vi "CC Create Script.vi"(11 "script name in":string) -> (3 "script name out":string)   [LabVIEW 2024]
uses:
  typedefs/CC cluster Exposure.ctl
  Detector/Detector Class/Detector enum Detector Integration Mode.ctl
  typedefs/CC cluster sidereal rate.ctl
  typedefs/CC Dithering.ctl
  typedefs/CC cluster Offset Dithering.ctl
  typedefs/CC Dithering Offsets.ctl
  typedefs/cc cluster muRA muDEC.ctl
  typedefs/CC cluster Random Dithering.ctl
  Detector/FITS/FITS enum Data Type.ctl
  Telescope/CC cluster Telescope Offsets.ctl
  typedefs/CC cluster Object.ctl
  typedefs/CC cluster RA and DEC.ctl
  Telescope/Telescope cluster Equinox.ctl
  Telescope/Telescope cluster Parallax.ctl
  Telescope/Telescope cluster Rotator.ctl
  Telescope/Telesope ring Frame.ctl
  typedefs/CC Script Step.ctl
  typedefs/CC enum Script Action.ctl
  Scripts/CC Rd Wr Script Creator Defaults.ctl
  typedefs/CC Dithering Map.ctl
  typedefs/CC enum Dithering Types.ctl
  Detector/FITS/FITS cluster Header Row.ctl
  typedefs/CC cluster Script.ctl
  Subsystems/SS typedef cluster Instrument Command Queue Data.ctl
  Scripts/CC Rd Wr Script Action.ctl
  Focus/Focus cluster MoveFocus Command Parameters.ctl
  typedefs/CC cluster Outlet Control.ctl
  typedefs/CC cluster Filter Wheel Parameters.ctl
  typedefs/CC cluster Acquire Parameters.ctl
  typedefs/CC cluster Pause Parameters.ctl
  Filter Wheel/Filter Wheel Object/Filter Wheel.lvclass
  Telescope/Telescope.lvclass
panel:
  in  "Script Path":path
  in  "Delete":bool
  in  "New Button":bool
  in  "Save As Button":bool
  in  "Script Name":u16(ring) items=["FocusScan_20231229_125359", "FocusScan_20240105_105553", "FocusScan_20240105_111439", "FocusScan_20240105_113950", "FocusScan_20240105_114731", "FocusScan_20240105_114814", "FocusScan_20240105_114924", "FocusScan_20240105_120012", "FocusScan_20240503_180609", "FocusScan_20240508_153210", "FocusScan_20240508_155921", "FocusScan_20240508_162716", "FocusScan_20240508_163450", "FocusScan_20240523_232945", "FocusScan_20240524_142601", "FocusScan_20240524_144640", "FocusScan_20240528_161613", "FocusScan_20240528_162302", "FocusScan_20240528_171448", "FocusScan_20240805_154542", "FocusScan_20240805_160317", "joe_test", "Obs_", "Obs_A00098", "Obs_A00099", "Obs_A00100", "Obs_A00101", "Obs_A00102", "Obs_A00103", "Obs_A00104", "Obs_A00105", "Obs_A00106", "Obs_A00107", "Obs_A00108", "Obs_A00109", "Obs_A00110", "Obs_A00111", "Obs_A00112", "Obs_A00113", "Obs_A00114", "Obs_A00115", "Obs_P00006", "Obs_P00008", "Obs_P00013", "Obs_P00014", "Obs_P00017", "Obs_P00018", "Obs_P00020", "Obs_P00022", "Obs_P00024", "Obs_P00025", "Obs_P00028", "Obs_P00033", "Obs_P00036", "Obs_P00037", "Obs_P00039", "Obs_P00040", "Obs_P00041", "Obs_P00042", "Obs_P00043", "Obs_P00044", "Obs_P00045", "Obs_P00046", "Obs_P00047", "Obs_P00049", "Obs_P00050", "Obs_P00051", "Obs_P00052", "Obs_P00053", "Obs_P00054", "Obs_P00055", "Obs_P00058", "Obs_P00059", "Obs_P00061", "Obs_P00064", "Obs_P00066", "Obs_P00067", "Obs_P00068", "Obs_P00069", "Obs_P00070", "Obs_P00071", "Obs_P00072", "Obs_P00073", "Obs_P00074", "Obs_P00075", "Obs_P00077", "Obs_P00078", "Obs_P00079", "Obs_P00080", "Obs_P00082", "Obs_P00083", "Obs_P00084", "Obs_P00085", "Obs_P00089", "Obs_P00090", "Obs_P00091", "Obs_P00092", "Obs_P00093", "Obs_P00094", "Obs_P00098", "Obs_P00099", "Obs_P00100", "Obs_P00101", "Obs_P00102", "Obs_P00103", "Obs_P00104", "Obs_P00105", "Obs_P00106", "Obs_P00107", "Obs_P00108", "Obs_P00109", "Obs_P00110", "Obs_P00111", "Obs_P00112", "Obs_P00113", "Obs_P00114", "Obs_P00115", "Obs_P00116", "Obs_P00117", "Obs_P00118", "Obs_P00119", "Obs_P00120", "Obs_P00121", "Obs_P00122", "Obs_P00123", "Obs_P00128", "Obs_P00129", "Obs_P00132", "Obs_P00133", "Obs_P00134", "Obs_P00135", "Obs_P00136", "Obs_P00137", "Obs_P00138", "Obs_P00139", "Obs_P00141", "Obs_P00142", "Obs_P00143", "Obs_P00144", "Obs_P00145", "Obs_P00146", "Obs_P00147", "Obs_P00148", "Obs_P00149", "Obs_P00150", "Obs_P00151", "Obs_P00152", "Obs_P00153", "Obs_P00162", "Obs_P00163", "Obs_P00164", "Obs_P00165", "Obs_P00166", "Obs_P00167", "Obs_P00168", "Obs_P00169", "Obs_P00170", "Obs_P00171", "Obs_P00172", "Obs_P00173", "Obs_P00174", "Obs_P00175", "Obs_P00176", "Obs_P00177", "Obs_P00178", "Obs_P00179", "Obs_P00180", "Obs_P00181", "Obs_P00182", "Obs_P00183", "Obs_P00184", "Obs_P00185", "Obs_P00186", "Obs_P00187", "Obs_P00188", "Obs_P00189", "Obs_P00190", "Obs_P00191", "Obs_P00192", "Obs_P00193", "Obs_P00194", "Obs_P00195", "Obs_P00196", "Obs_P00197", "Obs_P00198", "Obs_P00286", "Obs_P00287", "Obs_P00386", "Obs_P00387", "Obs_P00466", "Obs_P00467", "Obs_P00566", "Obs_P00567", "Obs_P00666", "Obs_P00667", "Obs_P00746", "Obs_P00747", "Obs_P00846", "Obs_P00847", "Obs_P00946", "Obs_P00947", "Obs_P01069", "Obs_P01070", "Obs_P01071", "Obs_P01666", "Obs_P01667", "power_test", "QuickObs_20231204_145334", "QuickObs_20231204_153100", "QuickObs_20231204_154938", "QuickObs_20231204_155404", "QuickObs_20231205_121758", "QuickObs_20240223_111256", "QuickObs_20240223_111314", "QuickObs_20240223_111324", "QuickObs_20240223_133303", "QuickObs_20240223_134117", "QuickObs_20240223_134543", "QuickObs_20240223_140340", "QuickObs_20240229_123536", "QuickObs_20240301_132858", "QuickObs_20240508_165728", "QuickObs_20240509_165826", "QuickObs_20240513_000104", "QuickObs_20240521_153751", "QuickObs_20240523_163529", "QuickObs_20240523_164254", "QuickObs_20240523_164316", "QuickObs_20240523_164354", "QuickObs_20240523_164558", "QuickObs_20240523_164836", "QuickObs_20240523_164937", "QuickObs_20240523_230241", "QuickObs_20240528_161057", "QuickObs_20240528_161742", "QuickObs_20240528_174732", "QuickObs_20240531_164244", "QuickObs_20240531_170220", "QuickObs_20240531_171735", "QuickObs_20240531_172457", "QuickObs_20240531_172609", "QuickObs_20240531_173041", "QuickObs_20240603_173837", "QuickObs_20240603_180156", "QuickObs_20240603_181309", "QuickObs_20240603_181617", "QuickObs_20240603_181820", "QuickObs_20240603_182118", "QuickObs_20240603_182553", "QuickObs_20240603_222300", "QuickObs_20240603_222614", "QuickObs_20240603_223000", "QuickObs_20240603_223344", "QuickObs_20240603_223915", "QuickObs_20240627_110641", "QuickObs_20240814_205941", "QuickObs_20240821_123647", "QuickObs_20240821_124152", "QuickObs_20240821_124547", "QuickObs_20240822_145236", "QuickObs_20240822_150150", "QuickObs_20240822_150414", "QuickObs_20240822_150607", "QuickObs_20240822_151545", "QuickObs_20240822_151844", "QuickObs_20240822_152439", "QuickObs_20240822_153207", "QuickObs_20240822_160035", "QuickObs_20240822_160608", "QuickObs_20240822_161129", "QuickObs_20240822_162300", "QuickObs_20240823_115930", "QuickObs_20240823_164127", "QuickObs_20240903_141058", "QuickObs_20240903_144343", "QuickObs_20240903_144643", "QuickObs_20240903_144654", "QuickObs_20240903_152244", "QuickObs_20240903_152705", "QuickObs_20240903_152922", "QuickObs_20240905_141101", "QuickObs_20240905_141629", "QuickObs_20240906_143746", "QuickObs_20240906_144857", "QuickObs_20240906_150256", "QuickObs_20240906_151102", "QuickObs_20240906_153044", "QuickObs_20240906_153745", "QuickObs_20240906_155352", "QuickObs_20240906_160445", "QuickObs_20240906_160908", "QuickObs_20240906_162122", "QuickObs_20240906_163123", "QuickObs_20240909_133034", "QuickObs_20240909_133716", "QuickObs_20240909_134628", "QuickObs_20240909_154242", "QuickObs_20240909_154542", "QuickObs_20240909_154633", "QuickObs_20240909_154947", "QuickObs_20240909_155344", "QuickObs_20240909_155456", "QuickObs_20240909_161838", "QuickObs_20240909_162303", "QuickObs_20240909_162501", "QuickObs_20240909_162628", "QuickObs_20240909_163134", "QuickObs_20240909_163322", "QuickObs_20240909_163424", "QuickObs_20240909_163636", "QuickObs_20240909_163836", "QuickObs_20240909_164419", "QuickObs_20240909_170410", "QuickObs_20240909_170734", "QuickObs_20240909_171023", "QuickObs_20240909_171530", "QuickObs_20240909_172951", "QuickObs_20240909_173144", "QuickObs_20240909_173940", "QuickObs_20240909_174042", "QuickObs_20240909_174245", "QuickObs_20240909_174431", "QuickObs_20240909_175227", "QuickObs_20240909_175352", "QuickObs_20240909_175611", "QuickObs_20240909_181046", "QuickObs_20240909_181216", "QuickObs_20240909_181334", "QuickObs_20240909_181505", "QuickObs_20240909_181623", "QuickObs_20240909_181711", "QuickObs_20240910_131018", "QuickObs_20240910_131144", "QuickObs_20240910_131417", "QuickObs_20240910_131600", "QuickObs_20240910_132017", "QuickObs_20240910_132419", "QuickObs_20240910_160952", "QuickObs_20240910_161811", "QuickObs_20240910_162606", "QuickObs_20240910_162747", "QuickObs_20240910_163442", "QuickObs_20240910_163715", "QuickObs_20240910_164302", "QuickObs_20240910_164445", "QuickObs_20240910_164629", "QuickObs_20240910_165143", "QuickObs_20240910_165430", "QuickObs_20240910_165827", "QuickObs_20240910_170042", "QuickObs_20240910_171946", "QuickObs_20240910_172143", "QuickObs_20240910_172830", "QuickObs_20240910_173047", "QuickObs_20240910_173807", "QuickObs_20240910_173956", "QuickObs_20240912_161641", "QuickObs_20240912_161849", "QuickObs_20240912_162058", "QuickObs_20240912_163325", "QuickObs_20240913_112043", "QuickObs_20240913_112810", "QuickObs_20240913_113523", "QuickObs_20240913_113948", "QuickObs_20240913_115247", "QuickObs_20240913_115435", "QuickObs_20240913_120048", "QuickObs_20240913_120152", "random", "Test Focus", "TestCommandLine"]
  in  "Save Script":bool
  in  "Close":bool
  in  "Script":i32(listbox)
  in  "Tab Control":T1(tab)
  in  "Units":string
  in  "Open Button":bool
  out "FITS Header Template":path
  in  "Save Header":bool
  in  "Add/Replace":bool
  in  "Comment":string
  in  "Value":string
  in  "Header Field":string(combo)
  in  "FITS Header":i32(listbox)
  in  "Type":T2
  in  "RA and DEC String":cluster{"RA":string, "DEC":string}={"RA"="HH:MM:SS.nnn", "DEC"="DEG:arcmin:arcsec.nn"} caption="RA and DEC"
  in  "Obj Add to Script":bool
  in  "Obj Remove":bool
  in  "Object Name":cluster{"Name":string}
  in  "Sidereal Rate":T3
  in  "Obj Add/Replace":bool
  in  "Objects":i32(listbox)
  in  "Proper Motion":T4
  in  "Offsets":T5
  in  "Exp Add to Script":bool
  in  "Exp Remove":bool
  in  "Exp Add/Replace":bool
  in  "Exposure":T6={"Mode"=enum."CDS", "Integration Time"=1.0, "Name"="", "Images"=1}
  in  "Exposures":i32(listbox)
  in  "Add FW 4":bool
  in  "Add FW 3":bool
  in  "Add FW 2":bool
  in  "Add FW 1":bool
  in  "Filter Wheel 4":i32(listbox)
  in  "Filter Wheel 3":i32(listbox)
  in  "Filter Wheel 2":i32(listbox) caption="FW HK"
  in  "Filter Wheel 1":i32(listbox) caption="FW YJ"
  in  "Name":string
  in  "Dither Add to Script":bool
  in  "Dithering Add/Replace":bool
  in  "Dithering":i32(listbox)
  in  "Dithering Remove":bool
  in  "Dither Select":enum32{"Random", "Offset"}(tab)
  in  "Random Dither":T8={"Count"=1, "Radius"=1.0, "Name"=""}
  in  "Dithering Offset":T9
  in  "Add Image Acq":bool
  in  "Acquire Parameters":T12
  in  "Add Macro":bool
  in  "Script to Call":u16(ring) items=["FocusScan_20231229_125359", "FocusScan_20240105_105553", "FocusScan_20240105_111439", "FocusScan_20240105_113950", "FocusScan_20240105_114731", "FocusScan_20240105_114814", "FocusScan_20240105_114924", "FocusScan_20240105_120012", "FocusScan_20240503_180609", "FocusScan_20240508_153210", "FocusScan_20240508_155921", "FocusScan_20240508_162716", "FocusScan_20240508_163450", "FocusScan_20240523_232945", "FocusScan_20240524_142601", "FocusScan_20240524_144640", "FocusScan_20240528_161613", "FocusScan_20240528_162302", "FocusScan_20240528_171448", "FocusScan_20240805_154542", "FocusScan_20240805_160317", "joe_test", "Obs_", "Obs_A00098", "Obs_A00099", "Obs_A00100", "Obs_A00101", "Obs_A00102", "Obs_A00103", "Obs_A00104", "Obs_A00105", "Obs_A00106", "Obs_A00107", "Obs_A00108", "Obs_A00109", "Obs_A00110", "Obs_A00111", "Obs_A00112", "Obs_A00113", "Obs_A00114", "Obs_A00115", "Obs_P00006", "Obs_P00008", "Obs_P00013", "Obs_P00014", "Obs_P00017", "Obs_P00018", "Obs_P00020", "Obs_P00022", "Obs_P00024", "Obs_P00025", "Obs_P00028", "Obs_P00033", "Obs_P00036", "Obs_P00037", "Obs_P00039", "Obs_P00040", "Obs_P00041", "Obs_P00042", "Obs_P00043", "Obs_P00044", "Obs_P00045", "Obs_P00046", "Obs_P00047", "Obs_P00049", "Obs_P00050", "Obs_P00051", "Obs_P00052", "Obs_P00053", "Obs_P00054", "Obs_P00055", "Obs_P00058", "Obs_P00059", "Obs_P00061", "Obs_P00064", "Obs_P00066", "Obs_P00067", "Obs_P00068", "Obs_P00069", "Obs_P00070", "Obs_P00071", "Obs_P00072", "Obs_P00073", "Obs_P00074", "Obs_P00075", "Obs_P00077", "Obs_P00078", "Obs_P00079", "Obs_P00080", "Obs_P00082", "Obs_P00083", "Obs_P00084", "Obs_P00085", "Obs_P00089", "Obs_P00090", "Obs_P00091", "Obs_P00092", "Obs_P00093", "Obs_P00094", "Obs_P00098", "Obs_P00099", "Obs_P00100", "Obs_P00101", "Obs_P00102", "Obs_P00103", "Obs_P00104", "Obs_P00105", "Obs_P00106", "Obs_P00107", "Obs_P00108", "Obs_P00109", "Obs_P00110", "Obs_P00111", "Obs_P00112", "Obs_P00113", "Obs_P00114", "Obs_P00115", "Obs_P00116", "Obs_P00117", "Obs_P00118", "Obs_P00119", "Obs_P00120", "Obs_P00121", "Obs_P00122", "Obs_P00123", "Obs_P00128", "Obs_P00129", "Obs_P00132", "Obs_P00133", "Obs_P00134", "Obs_P00135", "Obs_P00136", "Obs_P00137", "Obs_P00138", "Obs_P00139", "Obs_P00141", "Obs_P00142", "Obs_P00143", "Obs_P00144", "Obs_P00145", "Obs_P00146", "Obs_P00147", "Obs_P00148", "Obs_P00149", "Obs_P00150", "Obs_P00151", "Obs_P00152", "Obs_P00153", "Obs_P00162", "Obs_P00163", "Obs_P00164", "Obs_P00165", "Obs_P00166", "Obs_P00167", "Obs_P00168", "Obs_P00169", "Obs_P00170", "Obs_P00171", "Obs_P00172", "Obs_P00173", "Obs_P00174", "Obs_P00175", "Obs_P00176", "Obs_P00177", "Obs_P00178", "Obs_P00179", "Obs_P00180", "Obs_P00181", "Obs_P00182", "Obs_P00183", "Obs_P00184", "Obs_P00185", "Obs_P00186", "Obs_P00187", "Obs_P00188", "Obs_P00189", "Obs_P00190", "Obs_P00191", "Obs_P00192", "Obs_P00193", "Obs_P00194", "Obs_P00195", "Obs_P00196", "Obs_P00197", "Obs_P00198", "Obs_P00286", "Obs_P00287", "Obs_P00386", "Obs_P00387", "Obs_P00466", "Obs_P00467", "Obs_P00566", "Obs_P00567", "Obs_P00666", "Obs_P00667", "Obs_P00746", "Obs_P00747", "Obs_P00846", "Obs_P00847", "Obs_P00946", "Obs_P00947", "Obs_P01069", "Obs_P01070", "Obs_P01071", "Obs_P01666", "Obs_P01667", "power_test", "QuickObs_20231204_145334", "QuickObs_20231204_153100", "QuickObs_20231204_154938", "QuickObs_20231204_155404", "QuickObs_20231205_121758", "QuickObs_20240223_111256", "QuickObs_20240223_111314", "QuickObs_20240223_111324", "QuickObs_20240223_133303", "QuickObs_20240223_134117", "QuickObs_20240223_134543", "QuickObs_20240223_140340", "QuickObs_20240229_123536", "QuickObs_20240301_132858", "QuickObs_20240508_165728", "QuickObs_20240509_165826", "QuickObs_20240513_000104", "QuickObs_20240521_153751", "QuickObs_20240523_163529", "QuickObs_20240523_164254", "QuickObs_20240523_164316", "QuickObs_20240523_164354", "QuickObs_20240523_164558", "QuickObs_20240523_164836", "QuickObs_20240523_164937", "QuickObs_20240523_230241", "QuickObs_20240528_161057", "QuickObs_20240528_161742", "QuickObs_20240528_174732", "QuickObs_20240531_164244", "QuickObs_20240531_170220", "QuickObs_20240531_171735", "QuickObs_20240531_172457", "QuickObs_20240531_172609", "QuickObs_20240531_173041", "QuickObs_20240603_173837", "QuickObs_20240603_180156", "QuickObs_20240603_181309", "QuickObs_20240603_181617", "QuickObs_20240603_181820", "QuickObs_20240603_182118", "QuickObs_20240603_182553", "QuickObs_20240603_222300", "QuickObs_20240603_222614", "QuickObs_20240603_223000", "QuickObs_20240603_223344", "QuickObs_20240603_223915", "QuickObs_20240627_110641", "QuickObs_20240814_205941", "QuickObs_20240821_123647", "QuickObs_20240821_124152", "QuickObs_20240821_124547", "QuickObs_20240822_145236", "QuickObs_20240822_150150", "QuickObs_20240822_150414", "QuickObs_20240822_150607", "QuickObs_20240822_151545", "QuickObs_20240822_151844", "QuickObs_20240822_152439", "QuickObs_20240822_153207", "QuickObs_20240822_160035", "QuickObs_20240822_160608", "QuickObs_20240822_161129", "QuickObs_20240822_162300", "QuickObs_20240823_115930", "QuickObs_20240823_164127", "QuickObs_20240903_141058", "QuickObs_20240903_144343", "QuickObs_20240903_144643", "QuickObs_20240903_144654", "QuickObs_20240903_152244", "QuickObs_20240903_152705", "QuickObs_20240905_141101", "QuickObs_20240905_141629", "QuickObs_20240906_143746", "QuickObs_20240906_144857", "QuickObs_20240906_150256", "QuickObs_20240906_151102", "QuickObs_20240906_153044", "QuickObs_20240906_153745", "QuickObs_20240906_155352", "QuickObs_20240906_160445", "QuickObs_20240906_160908", "QuickObs_20240906_162122", "QuickObs_20240906_163123", "QuickObs_20240909_133034", "QuickObs_20240909_133716", "QuickObs_20240909_134628", "QuickObs_20240909_154242", "QuickObs_20240909_154542", "QuickObs_20240909_154633", "QuickObs_20240909_154947", "QuickObs_20240909_155344", "QuickObs_20240909_155456", "QuickObs_20240909_161838", "QuickObs_20240909_162303", "QuickObs_20240909_162501", "QuickObs_20240909_162628", "QuickObs_20240909_163134", "QuickObs_20240909_163322", "QuickObs_20240909_163424", "QuickObs_20240909_163636", "QuickObs_20240909_163836", "QuickObs_20240909_164419", "QuickObs_20240909_170410", "QuickObs_20240909_170734", "QuickObs_20240909_171023", "QuickObs_20240909_171530", "QuickObs_20240909_172951", "QuickObs_20240909_173144", "QuickObs_20240909_173940", "QuickObs_20240909_174042", "QuickObs_20240909_174245", "QuickObs_20240909_174431", "QuickObs_20240909_175227", "QuickObs_20240909_175352", "QuickObs_20240909_175611", "QuickObs_20240909_181046", "QuickObs_20240909_181216", "QuickObs_20240909_181334", "QuickObs_20240909_181505", "QuickObs_20240909_181623", "QuickObs_20240909_181711", "QuickObs_20240910_131018", "QuickObs_20240910_131144", "QuickObs_20240910_131417", "QuickObs_20240910_131600", "QuickObs_20240910_132017", "QuickObs_20240910_132419", "QuickObs_20240910_160952", "QuickObs_20240910_161811", "QuickObs_20240910_162606", "QuickObs_20240910_162747", "QuickObs_20240910_163442", "QuickObs_20240910_163715", "QuickObs_20240910_164302", "QuickObs_20240910_164445", "QuickObs_20240910_164629", "QuickObs_20240910_165143", "QuickObs_20240910_165430", "QuickObs_20240910_165827", "QuickObs_20240910_170042", "QuickObs_20240910_171946", "QuickObs_20240910_172143", "QuickObs_20240910_172830", "QuickObs_20240910_173047", "QuickObs_20240910_173807", "QuickObs_20240910_173956", "QuickObs_20240912_161641", "QuickObs_20240912_161849", "QuickObs_20240912_162058", "QuickObs_20240912_163325", "QuickObs_20240913_112043", "QuickObs_20240913_112810", "QuickObs_20240913_113523", "QuickObs_20240913_113948", "QuickObs_20240913_115247", "QuickObs_20240913_115435", "QuickObs_20240913_120048", "QuickObs_20240913_120152", "random", "Test Focus", "TestCommandLine"]
  in  "Move Telescope":bool
  in  "RA and DEC String 2":cluster{"RA":string, "DEC":string}={"RA"="HH:MM:SS.nnn", "DEC"="DEG:arcmin:arcsec.nn"} caption="RA and DEC"
  in  "Telescope Focus":T13
  in  "Message for User":string
  in  "Add Ask":bool caption="Add Ask to Script"
  in  "Seconds to Pause":dbl=10.0
  in  "Add Pause":bool caption="Add Pause to Script"
  in  "Home Focus":bool
  in  "Absolute":bool
  in  "Relative":bool
  in  "Steps":i32
  in  "Select Motor (0:n-1)":i32 min=0 max=3 step=1
  in  "Add Outlet Cmd":bool caption="Add Outlet Command Step"
  in  "Outlet State":bool
  in  "Outlet Index (0 based)":i32
  in  "Add CmdLine":bool caption="Add CmdLine to Script"
  in  "Command Line":string
  in  "Add No-op":bool caption="Add Noop to Script"
  out "Script As Text":string="DefineObject Alpha1234 Standard RA=123.456 DEC=456.789\nDefineExposure Number=1,Groups=1,ReadoutsPerGroup=1,TimeBetweenGroups=10,TimeBetweenReadouts=10\nDefineDithering DEC=0,-10,+10 RA=0,-10,+10\nMoveFilter A,B\nAcquireImages [This command acquires image at every dithering position]\n\n"
  in  "Send":bool
  in  "Script Line":string
  # "Select a Configuration (PRIME or RIMAS, FilterWheel, etc.)"
  # "\"\t   Y, J, or H can go with Open or Narrow only\n\"\t  Z must go with Open\n\"\t Dark can go with anything\n\"\t Open can go with anything\n\"\t Narrow can only go with T, J, H"
  # "arcseconds"
  # "arcseconds"
  # "Telescope Pointing"
  # "Focus"
  # "The noop command is used for testing purposes. There are no parameters."
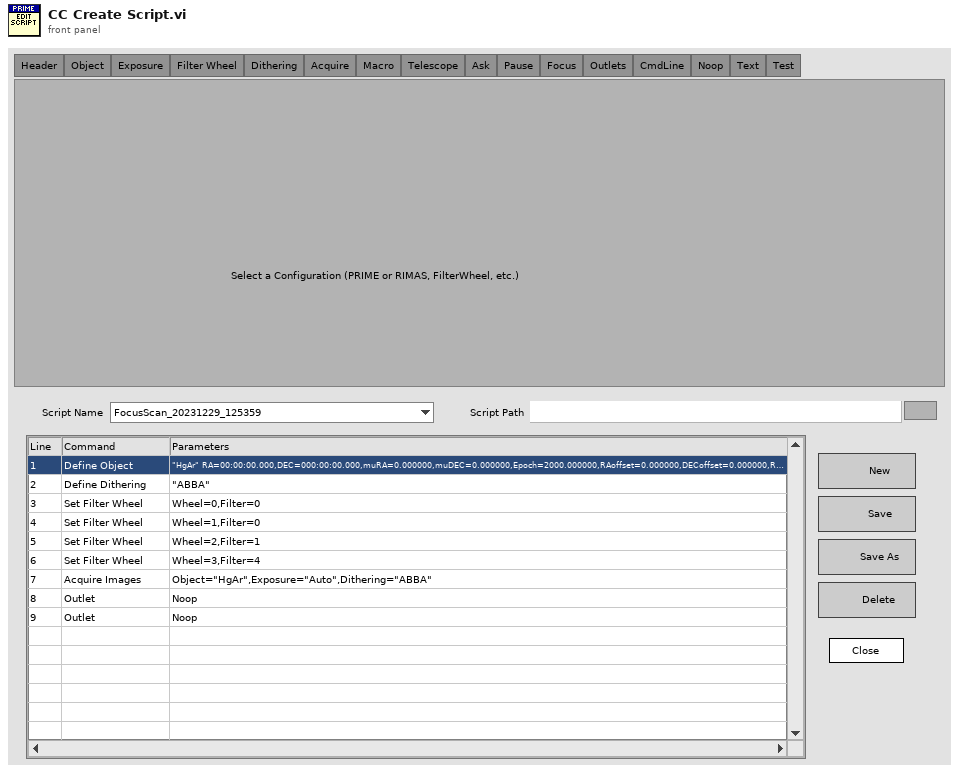
[diagram p1: front panel]
types:
  T1 = enum32{"Setup", "Header", "Object", "Exposure", "Filter Wheel", "Dithering", "Acquire", "Macro", "Telescope", "Ask", "Pause", "Focus", "Outlets", "CmdLine", "Noop", "Text", "Test"}
  T2 = typedef "FITS enum Data Type.ctl" = enum16{"String", "Integer", "Float"}
  T3 = typedef "CC cluster sidereal rate.ctl" = cluster{"dRA":dbl, "dDEC":dbl}
  T4 = typedef "cc cluster muRA muDEC.ctl" = cluster{"muRA":dbl, "muDEC":dbl, "Epoch":dbl}
  T5 = typedef "CC cluster Telescope Offsets.ctl" = cluster{"RA":dbl, "DEC":dbl, "ROT":dbl}
  T6 = typedef "CC cluster Exposure.ctl" = cluster{"Mode":T7, "Integration Time":dbl, "Name":string, "Images":i32}
  T7 = typedef "Detector enum Detector Integration Mode.ctl" = enum16{"Ramp", "CDS", "FOWLER2", "FOWLER4", "FOWLER8", "FOWLER16", "Raw"}
  T8 = typedef "CC cluster Random Dithering.ctl" = cluster{"Count":i32, "Radius":dbl, "Name":string}
  T9 = typedef "CC Dithering.ctl" = cluster{"Name":string, "Dithering Offsets":T10}
  T10 = typedef "CC cluster Offset Dithering.ctl" = cluster{"Offsets":T11[]}
  T11 = typedef "CC Dithering Offsets.ctl" = cluster{"DEC":dbl, "RA":dbl}
  T12 = cluster{"Object":string, "Exposure":string, "Dithering":string}
  T13 = cluster{"Focus Home":bool, "Move Focus":bool, "Position":dbl}
  T14 = typedef "CC cluster Object.ctl" = cluster{"Object":cluster{"Name":string}, "Sidereal Rate":T3, "RA and DEC":T15, "Proper Motion":T4, "Offsets":T5, "Equinox":T16, "Parallax":T17, "Rotator":T18, "Frame":T19, "Frac Rate":dbl, "Wavelength":dbl}
  T15 = typedef "CC cluster RA and DEC.ctl" = cluster{"RA":dbl, "DEC":dbl}
  T16 = typedef "Telescope cluster Equinox.ctl" = cluster{"Equinox Year":i32, "Equinox Prefix":string}
  T17 = typedef "Telescope cluster Parallax.ctl" = cluster{"Parallax":dbl, "rv kps":dbl}
  T18 = typedef "Telescope cluster Rotator.ctl" = cluster{"Frame":string, "PA":dbl}
  T19 = typedef "Telesope ring Frame.ctl" = enum16{"FK4", "FK5", "APPT", "GAPPT", "AZEL"}
  T20 = typedef "CC Script Step.ctl" = cluster{"Action":T21, "Data":variant}
  T21 = typedef "CC enum Script Action.ctl" = enum16{"Noop", "Define Object", "Define Exposure", "Define Dithering", "Acquire Images", "Set Filter Wheel", "Telescope Home", "Telescope Move", "Telescope RA DEC", "Focus Move Relative", "Focus Move Absolute", "Focus Set Home", "Macro", "Pause", "Ask User", "Define Random Dither", "CmdLine", "Outlet"}
  T22 = typedef "CC Rd Wr Script Creator Defaults.ctl" = cluster{"Script":string, "Script Path":path}
  T23 = typedef "CC Dithering Map.ctl" = cluster{"Name":string, "Dithering Offsets":T9, "Dithering Type":T24, "Random Dither":T8}
  T24 = typedef "CC enum Dithering Types.ctl" = enum16{"Random", "Offsets", "None"}
  T25 = typedef "FITS cluster Header Row.ctl" = cluster{"Field Name":string, "Type":T2, "Value":string, "Comment":string, "Units":string}
  T26 = cluster{"state":refnum<user-event>, "Object Map":map{string, T14}, "curr object":string, "Exp Map":map{string, T6}, "Script":T20[], "Settings":T22, "test":T20[], "Dither Map":map{string, T23}, "Hdr Map":map{string, T25}}
  T27 = typedef "CC cluster Script.ctl" = cluster{"Name":string, "Script":T20[]}
  T28 = typedef "CC Rd Wr Script Action.ctl" = enum16{"Read", "Write", "List", "Delete"}
  T29 = typedef "SS typedef cluster Instrument Command Queue Data.ctl" = cluster{"Cmd":string, "Parameters":variant}
  T30 = typedef "Focus cluster MoveFocus Command Parameters.ctl" = cluster{"Motor":i32, "Position":i32}
  T31 = typedef "CC cluster Outlet Control.ctl" = cluster{"Outlet Idx":i32, "State":bool}
  T32 = typedef "CC cluster Filter Wheel Parameters.ctl" = cluster{"Wheel":i32, "Filter":i32}
  T33 = enum32{"Setup", "Object", "Exposure", "Dithering", "Acquire", "Filter Wheel", "Focus", "Macro", "Ask", "Pause", "Noop", "Text", "Test"}
  T34 = enum32{"Setup", "Object", "Exposure", "Dithering", "Acquire", "Filter Wheel", "Focus", "Ask", "Pause", "Noop", "Text", "Test"}
  T35 = typedef "CC cluster Acquire Parameters.ctl" = cluster{"Object":string, "Exposure":string, "Dithering":string}
  T36 = enum32{"Setup", "Object", "Exposure", "Filter Wheel", "Dithering", "Acquire", "Macro", "Telescope", "Ask", "Pause", "PicoMotors", "Noop", "Text", "Test"}
  T37 = typedef "CC cluster Pause Parameters.ctl" = cluster{"Time (s)":dbl}
  T38 = enum32{"Setup", "Header Info", "Object", "Exposure", "Filter Wheel", "Dithering", "Acquire", "Macro", "Telescope", "Ask", "Pause", "Focus Motors", "Noop", "Text", "Test"}
  T39 = typedef "CC cluster Script Panel Defaults.ctl" = cluster{"Script Name":string, "Script Path":path}
  T40 = typedef "RIMAS Detector Config.ctl" = cluster{"Detector":u16, "Offsets":u16[][], "Detector Computer":T41, "FITS hdr template0":path, "FITS hdr template1":path, "FITS Data File Path":path, "FITS Detector Settings":T42, "Sim Folder":path, "Integration Mode":T7, "Integration Time":dbl, "Frame Int Time":dbl}
  T41 = typedef "RIMAS Detector Server Config.ctl" = cluster{"Machine":string, "Password":string, "FITS File Path":string, "Port":u16, "Header Path":string, "Name":string}
  T42 = typedef "RIMAS Observation Config.ctl" = cluster{"Exp Time Short":dbl, "# of Frames":dbl, "Exp Time Long":dbl, "# of Groups":dbl, "Object Name":string, "Object":string, "Obs Type":string, "Image Type":string, "Observer":string, "Observer Affiliation":string}
  T43 = typedef "CC cluster Hardware Config.ctl" = cluster{"Installed Hardware":T44[]}
  T44 = typedef "CC cluster Device Index.ctl" = cluster{"Device Type Name":string, "Curr Device Name":string, "All Instances":string[]}
  T45 = typedef "Filter Wheel.lvclass/Filter Wheel configuration.ctl" = cluster{"Num Wheels":i32, "Filters":T46[], "Invalid Combinations":i32[][], "Addr":refnum<visa-resource-name>, "Name":string, "Simulate":bool, "Default Speed":u16, "Homing":T47[]}
  T46 = typedef "Filter Wheel.lvclass/Filter Wheel Details.ctl" = cluster{"Names":string[], "Relative Position":i32[], "Wheel Name":string, "Size":i32}
  T47 = typedef "Filter Wheel Arduino Homing cluster.ctl" = cluster{"Direction":bool, "Speed":i32, "Accel":i32, "Error Cnts":i32, "Homing Delta":i32}
  T48 = typedef "LVPoint32TypeDef.ctl" = cluster{"Horizontal":i32, "Vertical":i32}
  T49 = typedef "LVRowAndColumnTypeDef.ctl" = cluster{"Row":i32, "Column":i32}
  T50 = enum32{"Setup", "Object", "Exposure", "Dithering", "Acquire", "Filter Wheel", "Ask", "Pause", "Noop", "Text"}
  T51 = enum32{"Setup", "Header Info", "Object", "Exposure", "Filter Wheel", "Dithering", "Acquire", "Macro", "Telescope", "Ask", "Pause", "PicoMotors", "Noop", "Text", "Test"}
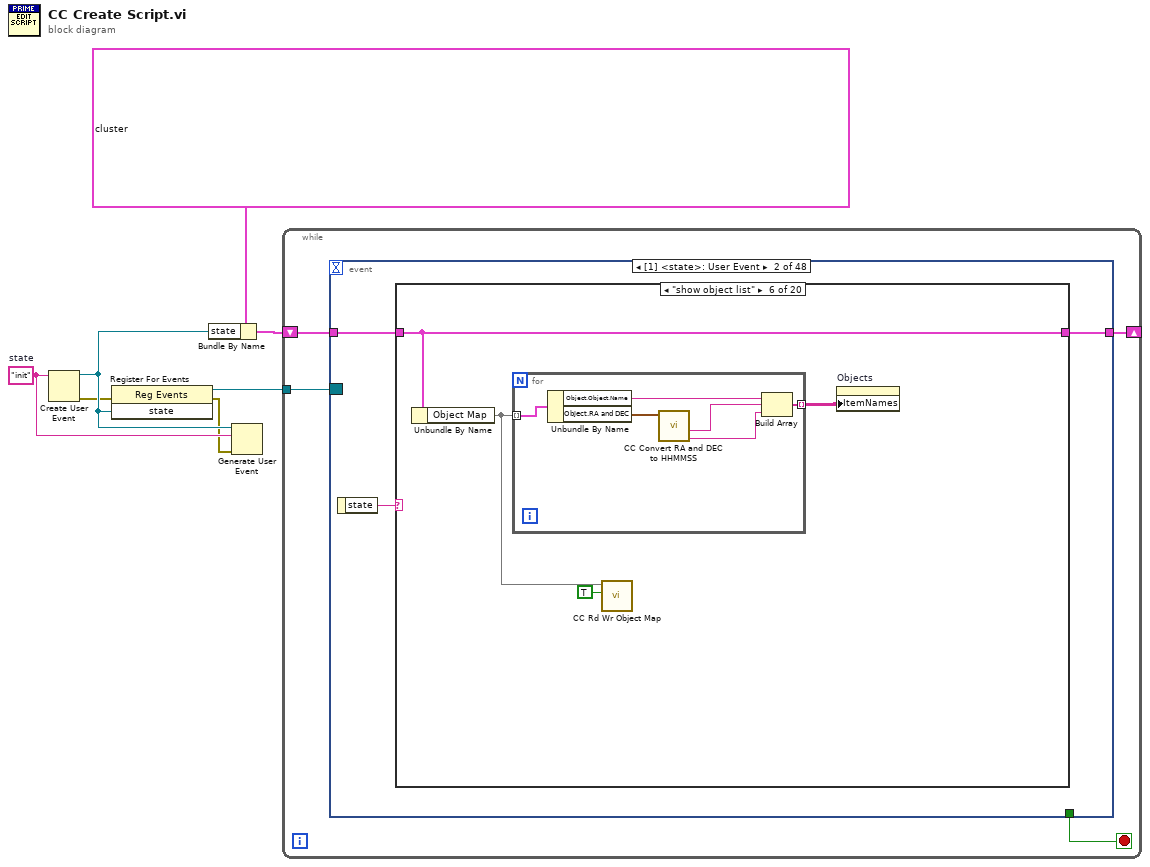
[diagram p0: block diagram]
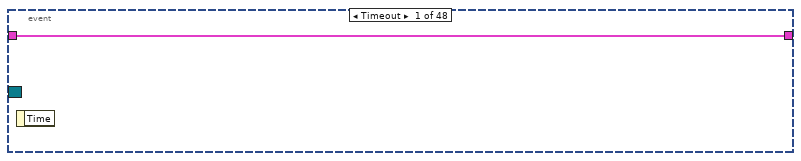
[diagram p2: hidden frame]
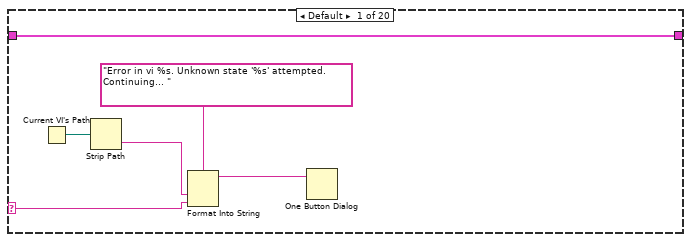
[diagram p3: hidden frame]
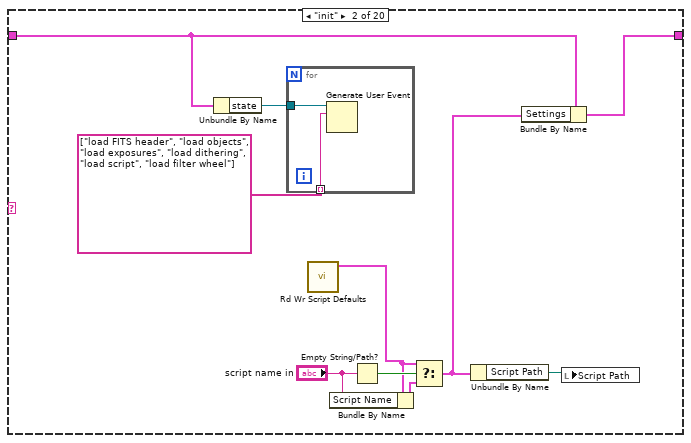
[diagram p4: hidden frame]
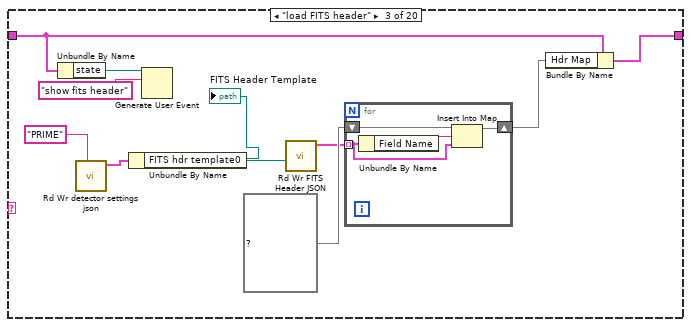
[diagram p5: hidden frame]
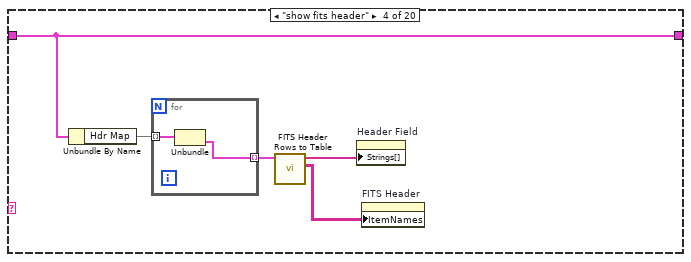
[diagram p6: hidden frame]
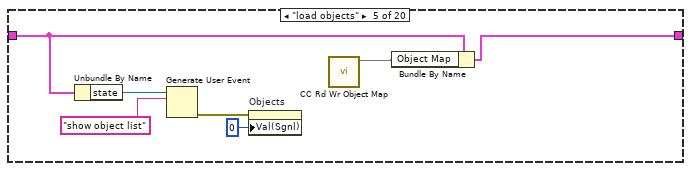
[diagram p7: hidden frame]
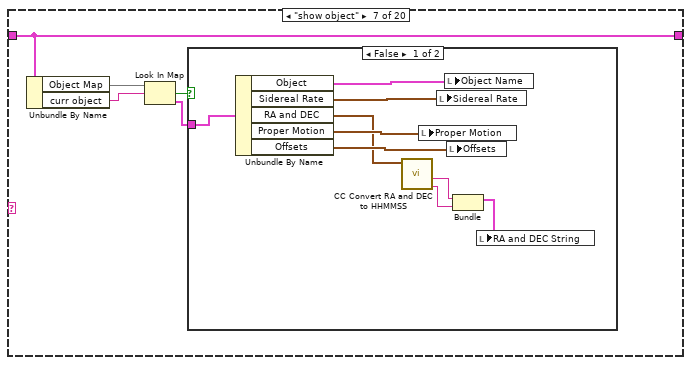
[diagram p8: hidden frame]
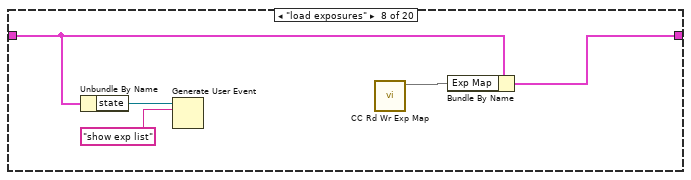
[diagram p10: hidden frame]
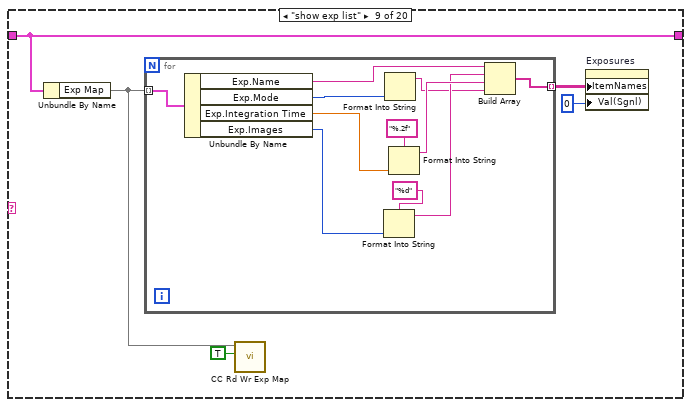
[diagram p11: hidden frame]
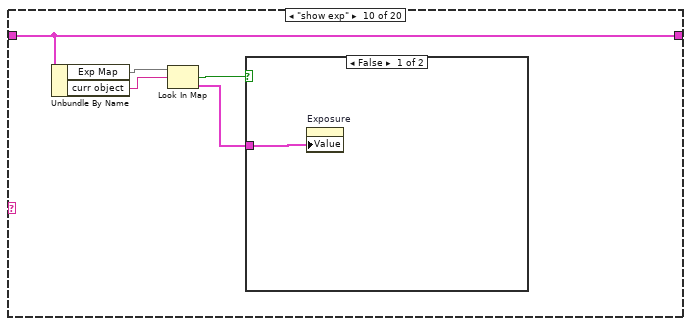
[diagram p12: hidden frame]
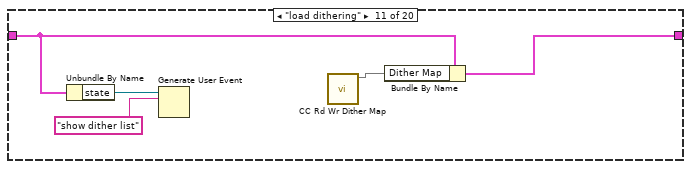
[diagram p14: hidden frame]
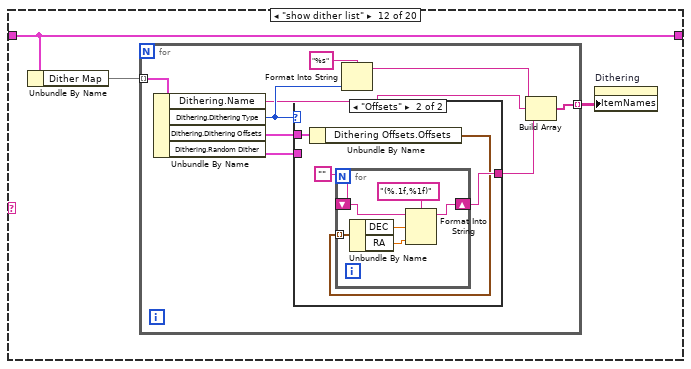
[diagram p15: hidden frame]
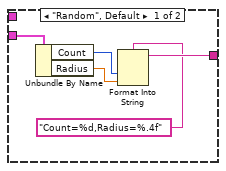
[diagram p16: hidden frame]
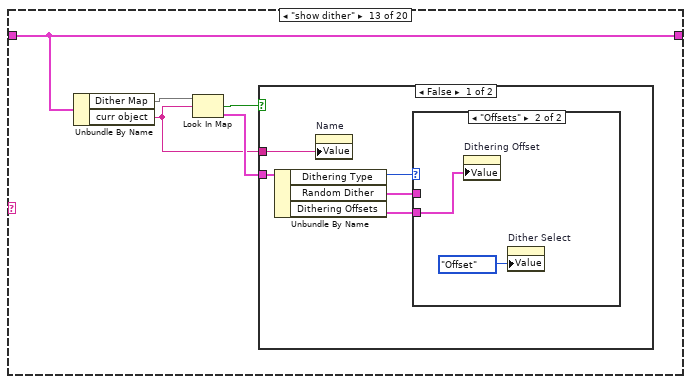
[diagram p17: hidden frame]
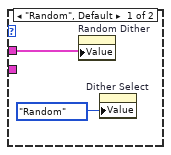
[diagram p18: hidden frame]
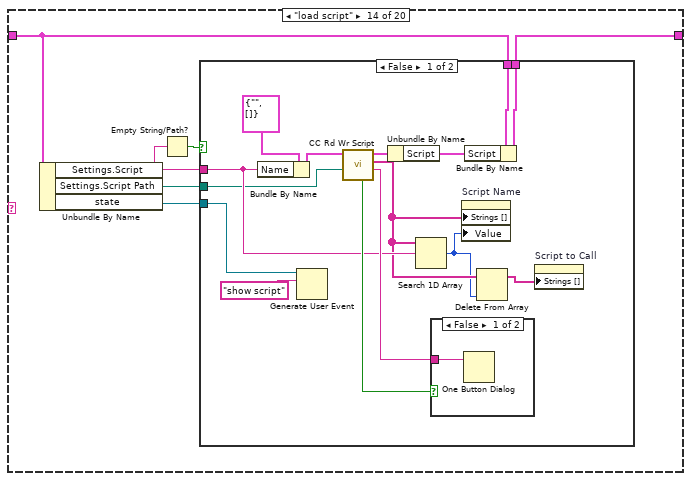
[diagram p20: hidden frame]
diagram:
  w3 = "init"  # state
  n1 = Create User Event(user event datatype=w3) -> (user event=w5:refnum<user-event>, error out=w1:errorcluster)  [unwired: 1 in]
  n2 = register-events(error in=w1, w5) -> (reference out=w4:refnum<event-registration>, error out=w2:errorcluster)  [unwired: 1 in]
  n3 = Bundle By Name(cluster=T26 {"state"=refnum, "Object Map"={}, "curr object"="", "Exp Map"={}, "Script"=[], "Settings"={"Script"="", "Script Path"=path ""}, "test"=[], "Dither Map"={}, "Hdr Map"={}}, "state"=w5) -> (w6:T26)
  n4 = Generate User Event(user event=w5, event data cluster=w3, error in=w2) -> ()  [unwired: 1 in, 2 out]
  n5 = while {
    tunnel: w4 -> [w11]
    shift-right: [w9] -> _
    shift-left: w6 -> [w10]
    stop <- w8 stop-if-true
    n6 = event shown="[1] <state>: User Event" {
      selector: w11 -> [_ _ _ _ _ _ _ _ _ _ _ _ _ _ _ _ _ _ _ _ _ _ _ _ _ _ _ _ _ _ _ _ _ _ _ _ _ _ _ _ _ _ _ _ _ _ _ _]
      dyn-events: _ -> [_ _ _ _ _ _ _ _ _ _ _ _ _ _ _ _ _ _ _ _ _ _ _ _ _ _ _ _ _ _ _ _ _ _ _ _ _ _ _ _ _ _ _ _ _ _ _ _]
      timeout: _ -> [_ _ _ _ _ _ _ _ _ _ _ _ _ _ _ _ _ _ _ _ _ _ _ _ _ _ _ _ _ _ _ _ _ _ _ _ _ _ _ _ _ _ _ _ _ _ _ _]
      tunnel: w10 -> [w12 w14 w271 w283 w285 w288 w310 w324 w328 w339 w341 w352 w365 w386 w392 w403 w415 w425 w445 w460 w483 w508 w539 w550 w556 w571 w585 w622 w628 w649 w688 w699 w711 w716 w727 w733 w741 w792 w901 w915 w926 w938 w947 w959 w974 w976 w1010 w1014]
      tunnel: [w12 w13 w272 w283 w285 w289 w310 w324 w328 w336 w342 w353 w366 w387 w390 w404 w416 w426 w446 w459 w482 w507 w540 w551 w557 w572 w586 w623 w627 w649 w689 w700 w711 w715 w727 w734 w741 w791 w902 w916 w927 w939 w948 w960 w974 w975 w1010 w1014] -> w9
      tunnel: [_ _ _ _ _ _ _ _ _ _ _ _ _ _ _ _ _ _ _ _ _ _ _ _ _ _ _ _ _ _ _ _ _ _ _ _ _ _ _ _ _ _ _ _ _ _ _ "Close"] -> w8
      event Timeout {
        n7 = event-data() -> ()  [unwired: 1 in, 1 out]
      }
      event User Event {
        n8 = event-data() -> ("state"=w15:string)  [unwired: 1 in]
        n9 = case shown="\"show object list\"" w15 {
          selector: w15 -> [w20 _ _ _ _ _ _ _ _ _ _ _ _ _ _ _ _ _ _ _]
          tunnel: w14 -> [w16 w28 w36 w50 w59 w64 w76 w86 w95 w111 w114 w120 w146 w163 w202 w230 w235 w250 w255 w258]
          tunnel: [w16 w29 w41 w50 w61 w64 w76 w89 w95 w111 w117 w120 w146 w164 w202 w230 w235 w250 w255 w258] -> w13
          frame Default {
            n10 = Current VI's Path() -> (path=w19:path)
            n11 = Strip Path(path=w19) -> (name=w18:string)  [unwired: 1 out]
            n12 = Format Into String(format string="Error in vi %s. Unknown state '%s' attempted. Continuing... ", w18, w20) -> (resulting string=w17:string)  [unwired: 2 in, 1 out]
            n13 = One Button Dialog(message=w17) -> ()  [unwired: 1 in, 1 out]
          }
          frame "init" {
            n14 = Unbundle By Name(w28) -> ("state"=w31:refnum<user-event>)
            n15 = for {
              tunnel: w31 -> [w33]
              tunnel: string[] ["load FITS header", "load objects", "load exposures", "load dithering", "load script", "load filter wheel"] -> [w32] mode=indexing
              n16 = Generate User Event(user event=w33, event data cluster=w32) -> ()  [unwired: 2 in, 2 out]
            }
            n17 = call "Rd Wr Script Defaults.vi"() -> ("Script Settings"=w22:T39)  [unwired: 10 in, 1 out]
            n18 = Bundle By Name(cluster=w22, "Script Name"="script name in") -> (w25:T39)
            n19 = Empty String/Path?(string/path="script name in") -> (empty?=w27:bool)
            n20 = Select(t=w22, s=w27, f=w25) -> (s? t:f=w23:T39)
            n21 = Unbundle By Name(w23) -> ("Script Path"=w24:path)
            n22 = Bundle By Name(cluster=w28, "Settings"=w23) -> (w29:T26)
            n23 = local write "Script Path"(w24) -> ()
          }
          frame "load FITS header" {
            n24 = Unbundle By Name(w36) -> ("state"=w35:refnum<user-event>)
            n25 = call "Rd Wr detector settings json.vi"("Detector Name"="PRIME") -> ("Detector Config"=w42:T40)  [unwired: 9 in, 1 out]
            n26 = Unbundle By Name(w42) -> ("FITS hdr template0"=w40:path)
            "FITS Header Template" <- w40
            n27 = Generate User Event(user event=w35, event data cluster="show fits header" ("event data")) -> ()  [unwired: 2 in, 2 out]
            n28 = call "Rd Wr FITS Header JSON.vi"("FITS Template"=w40) -> ("FITS Hdr Rows"=w37:T25[])  [unwired: 9 in, 1 out]
            n29 = for {
              tunnel: w37 -> [w45] mode=indexing
              shift-right: [w44] -> w38
              shift-left: map{string, T25} {} ("Hdr Map") -> [w47]
              n30 = Unbundle By Name(w45) -> ("Field Name"=w46:string)
              n31 = Insert Into Map(map in=w47, key=w46, value=w45) -> (map out=w44:map{string, T25})  [unwired: 2 out]
            }
            n32 = Bundle By Name(cluster=w36, "Hdr Map"=w38) -> (w41:T26)
          }
          frame "show fits header" {
            n33 = Unbundle By Name(w50) -> ("Hdr Map"=w49:map{string, T25})
            n34 = for {
              tunnel: w49 -> [w54] mode=indexing
              tunnel: [w53] -> w48 mode=indexing
              n35 = Unbundle(w54) -> (w53:T25)  [unwired: 1 out]
            }
            n36 = call "FITS Header Rows to Table.vi"("FITS Hdr Rows"=w48) -> ("table"=w51:string[][], "Keywords"=w52:string[])  [unwired: 9 in]
            n37 = property on="Header Field" class="CmbBox"("Strings[]"=w52) -> ()  [unwired: 2 in, 2 out]
            n38 = property on="FITS Header" class="MCListbox (strict)"("ItemNames"=w51) -> ()  [unwired: 2 in, 2 out]
          }
          frame "load objects" {
            n39 = Unbundle By Name(w59) -> ("state"=w58:refnum<user-event>)
            n40 = Generate User Event(user event=w58, event data cluster="show object list" ("event data")) -> (error out=w56:errorcluster)  [unwired: 2 in, 1 out]
            n41 = property on="Objects" class="MCListbox (strict)"(error in=w56, "Val(Sgnl)"=0 ("Value (Signaling)")) -> ()  [unwired: 1 in, 2 out]
            n42 = call "CC Rd Wr Object Map.vi"() -> ("Object Map in"=w60:map{string, T14})  [unwired: 10 in, 1 out]
            n43 = Bundle By Name(cluster=w59, "Object Map"=w60) -> (w61:T26)
          }
          frame "show object list" {
            n44 = Unbundle By Name(w64) -> ("Object Map"=w63:map{string, T14})
            n45 = for {
              tunnel: w63 -> [w71] mode=indexing
              tunnel: [w69] -> w65 mode=indexing
              n46 = Unbundle By Name(w71) -> ("Object.Object.Name"=w70:string, "Object.RA and DEC"=w68:T15)
              n47 = call "CC Convert RA and DEC to HHMMSS.vi"("RA and DEC"=w68) -> ("DEC String"=w66:string, "RA String"=w67:string)  [unwired: 7 in, 2 out]
              n48 = Build Array(w70, w67, w66) -> (w69:string[])
            }
            n49 = call "CC Rd Wr Object Map.vi"("Write? (F:Read)"=TRUE, "Object Map in"=w63) -> ()  [unwired: 8 in, 2 out]
            n50 = property on="Objects" class="MCListbox (strict)"("ItemNames"=w65) -> ()  [unwired: 2 in, 2 out]
          }
          frame "show object" {
            n51 = Unbundle By Name(w76) -> ("Object Map"=w75:map{string, T14}, "curr object"=w74:string)
            n52 = Look In Map(map=w75, key=w74) -> (key not found?=w73:bool, value=w72:T14)  [unwired: 1 in]
            n53 = case shown="False" w73 {
              tunnel: w72 -> [w85 _]
              frame False {
                n54 = Unbundle By Name(w85) -> ("Object"=w84:cluster{"Name":string}, "Sidereal Rate"=w83:T3, "RA and DEC"=w80:T15, "Proper Motion"=w82:T4, "Offsets"=w81:T5)
                n55 = call "CC Convert RA and DEC to HHMMSS.vi"("RA and DEC"=w80) -> ("DEC String"=w78:string, "RA String"=w79:string)  [unwired: 7 in, 2 out]
                n56 = local write "Proper Motion"(w82) -> ()
                n57 = local write "Sidereal Rate"(w83) -> ()
                n58 = local write "Object Name"(w84) -> ()
                n59 = local write "Offsets"(w81) -> ()
                n60 = Bundle("RA String"=w79, "DEC String"=w78) -> (w77:cluster{"RA String":string, "DEC String":string})  [unwired: 1 in]
                n61 = local write "RA and DEC String"(w77) -> ()
              }
              frame True {
              }
            }
          }
          frame "load exposures" {
            n62 = Unbundle By Name(w86) -> ("state"=w88:refnum<user-event>)
            n63 = Generate User Event(user event=w88, event data cluster="show exp list" ("event data")) -> ()  [unwired: 2 in, 2 out]
            n64 = call "CC Rd Wr Exp Map.vi"() -> ("Exp Map"=w90:map{string, T6})  [unwired: 10 in, 1 out]
            n65 = Bundle By Name(cluster=w86, "Exp Map"=w90) -> (w89:T26)
          }
          frame "show exp list" {
            n66 = Unbundle By Name(w95) -> ("Exp Map"=w93:map{string, T6})
            n67 = for {
              tunnel: w93 -> [w106] mode=indexing
              tunnel: [w102] -> w94 mode=indexing
              n68 = Unbundle By Name(w106) -> ("Exp.Name"=w105:string, "Exp.Mode"=w104:T7, "Exp.Integration Time"=w101:dbl, "Exp.Images"=w99:i32)
              n69 = Format Into String(format string="%d", w99) -> (resulting string=w97:string)  [unwired: 2 in, 1 out]
              n70 = Format Into String(w104) -> (resulting string=w96:string)  [unwired: 3 in, 1 out]
              n71 = Format Into String(format string="%.2f", w101) -> (resulting string=w100:string)  [unwired: 2 in, 1 out]
              n72 = Build Array(w105, w97, w100, w96) -> (w102:string[])
            }
            n73 = call "CC Rd Wr Exp Map.vi"("Write? (F:Read)"=TRUE, "Exp Map"=w93) -> ()  [unwired: 8 in, 2 out]
            n74 = property on="Exposures" class="MCListbox (strict)"("ItemNames"=w94, "Val(Sgnl)"=0 ("Value (Signaling)")) -> ()  [unwired: 2 in, 2 out]
          }
          frame "show exp" {
            n75 = Unbundle By Name(w111) -> ("Exp Map"=w110:map{string, T6}, "curr object"=w109:string)
            n76 = Look In Map(map=w110, key=w109) -> (key not found?=w108:bool, value=w107:T6)  [unwired: 1 in]
            n77 = case shown="False" w108 {
              tunnel: w107 -> [w112 _]
              frame False {
                n78 = property on="Exposure" class="Clust (strict)"("Value"=w112) -> ()  [unwired: 2 in, 2 out]
              }
              frame True {
              }
            }
          }
          frame "load dithering" {
            n79 = Unbundle By Name(w114) -> ("state"=w116:refnum<user-event>)
            n80 = Generate User Event(user event=w116, event data cluster="show dither list" ("event data")) -> ()  [unwired: 2 in, 2 out]
            n81 = call "CC Rd Wr Dither Map.vi"() -> ("Dither Map"=w113:map{string, T23})  [unwired: 10 in, 1 out]
            n82 = Bundle By Name(cluster=w114, "Dither Map"=w113) -> (w117:T26)
          }
          frame "show dither list" {
            n83 = Unbundle By Name(w120) -> ("Dither Map"=w118:map{string, T23})
            n84 = for {
              tunnel: w118 -> [w129] mode=indexing
              tunnel: [w126] -> w119 mode=indexing
              n85 = Unbundle By Name(w129) -> ("Dithering.Name"=w121:string, "Dithering.Dithering Type"=w123:T24, "Dithering.Dithering Offsets"=w128:T9, "Dithering.Random Dither"=w122:T8)
              n86 = case shown="\"Offsets\"" w123 {
                tunnel: w128 -> [_ w136]
                tunnel: [w131 w137] -> w127
                tunnel: w122 -> [w134 _]
                frame "Random", Default {
                  n87 = Unbundle By Name(w134) -> ("Count"=w133:i32, "Radius"=w132:dbl)
                  n88 = Format Into String(format string="Count=%d,Radius=%.4f", w133, w132) -> (resulting string=w131:string)  [unwired: 2 in, 1 out]
                }
                frame "Offsets" {
                  n89 = Unbundle By Name(w136) -> ("Dithering Offsets.Offsets"=w135:T11[])
                  n90 = for {
                    tunnel: w135 -> [w143] mode=indexing
                    shift-right: [w139] -> w137
                    shift-left: "" -> [w140]
                    n91 = Unbundle By Name(w143) -> ("DEC"=w142:dbl, "RA"=w141:dbl)
                    n92 = Format Into String(format string="(%.1f,%1f)", initial string=w140, w142, w141) -> (resulting string=w139:string)  [unwired: 1 in, 1 out]
                  }
                }
              }
              n93 = Format Into String(format string="%s", w123) -> (resulting string=w124:string)  [unwired: 2 in, 1 out]
              n94 = Build Array(w124, w121, w127) -> (w126:string[])
            }
            n95 = property on="Dithering" class="MCListbox (strict)"("ItemNames"=w119) -> ()  [unwired: 2 in, 2 out]
          }
          frame "show dither" {
            n96 = Unbundle By Name(w146) -> ("Dither Map"=w149:map{string, T23}, "curr object"=w145:string)
            n97 = Look In Map(map=w149, key=w145) -> (key not found?=w148:bool, value=w147:T23)  [unwired: 1 in]
            n98 = case shown="False" w148 {
              tunnel: w147 -> [w154 _]
              tunnel: w145 -> [w150 _]
              frame False {
                n99 = Unbundle By Name(w154) -> ("Dithering Type"=w153:T24, "Random Dither"=w151:T8, "Dithering Offsets"=w152:T9)
                n100 = property on="Name" class="Str"("Value"=w150) -> ()  [unwired: 2 in, 2 out]
                n101 = case shown="\"Offsets\"" w153 {
                  tunnel: w152 -> [_ w158]
                  tunnel: w151 -> [w156 _]
                  frame "Random", Default {
                    n102 = property on="Random Dither" class="Clust (strict)"("Value"=w156) -> ()  [unwired: 2 in, 2 out]
                    n103 = property on="Dither Select" class="TabCtl (strict)"("Value"=enum32{"Random", "Offset"}."Random" ("Dither Select")) -> ()  [unwired: 2 in, 2 out]
                  }
                  frame "Offsets" {
                    n104 = property on="Dithering Offset" class="Clust (strict)"("Value"=w158) -> ()  [unwired: 2 in, 2 out]
                    n105 = property on="Dither Select" class="TabCtl (strict)"("Value"=enum32{"Random", "Offset"}."Offset" ("Dither Select")) -> ()  [unwired: 2 in, 2 out]
                  }
                }
              }
              frame True {
              }
            }
          }
          frame "load script" {
            n106 = Unbundle By Name(w163) -> ("Settings.Script"=w161:string, "Settings.Script Path"=w159:path, "state"=w162:refnum<user-event>)
            n107 = Empty String/Path?(string/path=w161) -> (empty?=w160:bool)
            n108 = case shown="False" w160 {
              tunnel: [w175 w182] -> w164
              tunnel: w163 -> [w174 w182]
              tunnel: w162 -> [w173 _]
              tunnel: w161 -> [w169 _]
              tunnel: w159 -> [w165 _]
              frame False {
                n109 = Bundle By Name(cluster=T27 {"Name"="", "Script"=[]} ("Script"), "Name"=w169) -> (w178:T27)
                n110 = Generate User Event(user event=w173, event data cluster="show script" ("event data")) -> ()  [unwired: 2 in, 2 out]
                n111 = call "CC Rd Wr Script.vi"("Script Path"=w165, "Script"=w178) -> ("Syntax Errors"=w170:string, "Script List"=w168:string[], "Script"=w177:T27, "Script Ok?"=w171:bool)  [unwired: 4 in, 2 out]
                n112 = Unbundle By Name(w177) -> ("Script"=w176:T20[])
                n113 = Search 1D Array(1D array=w168, element=w169) -> (index of element=w167:i32)  [unwired: 1 in]
                n114 = case shown="False" w171 {
                  tunnel: w170 -> [w180 _]
                  frame False {
                    n115 = One Button Dialog(message=w180) -> ()  [unwired: 1 in, 1 out]
                  }
                  frame True {
                  }
                }
                n116 = property on="Script Name" class="Ring (strict)"("Strings []"=w168, "Value"=w167) -> ()  [unwired: 2 in, 2 out]
                n117 = Bundle By Name(cluster=w174, "Script"=w176) -> (w175:T26)
                n118 = Delete From Array(array=w168, index=w167) -> (array with subset deleted=w166:string[])  [unwired: 1 in, 1 out]
                n119 = property on="Script to Call" class="Ring (strict)"("Strings []"=w166) -> ()  [unwired: 2 in, 2 out]
              }
              frame True {
                n120 = property on="Script" class="MCListbox (strict)"("ItemNames"=string[][] [] ("Item Names")) -> ()  [unwired: 2 in, 2 out]
              }
            }
          }
          frame "load filter wheel" {
            n121 = call "CC Rd Wr Hardware Configuration.vi"() -> ("Hardware Config out"=w185:T43)  [unwired: 8 in, 3 out]
            n122 = control-ref of="Filter Wheel 4"() -> (w197:refnum<vi>)
            n123 = control-ref of="Add FW 1"() -> (w192:refnum<vi>)
            n124 = control-ref of="Add FW 2"() -> (w189:refnum<vi>)
            n125 = control-ref of="Add FW 3"() -> (w190:refnum<vi>)
            n126 = control-ref of="Add FW 4"() -> (w191:refnum<vi>)
            n127 = control-ref of="Filter Wheel 3"() -> (w198:refnum<vi>)
            n128 = control-ref of="Filter Wheel 2"() -> (w199:refnum<vi>)
            n129 = control-ref of="Filter Wheel 1"() -> (w200:refnum<vi>)
            n130 = Unbundle By Name(w185) -> ("Installed Hardware"=w184:T44[])
            n131 = Build Array(w192, w189, w190, w191) -> (w188:refnum<vi>[])
            n132 = Build Array(w200, w199, w198, w197) -> (w193:refnum<vi>[])
            n133 = call "CC Get Current Device.vi"("Device Type Name"="filter wheel", "Hardware.Installed Hardware"=w184) -> ("Curr Device Name"=w183:string)  [unwired: 7 in, 2 out]
            n134 = for {
              tunnel: [w208] -> w194 mode=indexing
              tunnel: w193 -> [w207] mode=indexing
              tunnel: w188 -> [w205] mode=indexing
              tunnel: [w203] -> w187 mode=indexing
              n135 = property class="LstBox (strict)"(reference=w207, "Visible"=FALSE) -> (reference out=w208:refnum<vi>)  [unwired: 1 in, 1 out]
              n136 = property class="Bool"(reference=w205, "Visible"=FALSE) -> (reference out=w203:refnum<vi>)  [unwired: 1 in, 1 out]
            }
            n137 = call "Rd Wr Filter Wheel Settings.vi"("Wheel Name"=w183) -> ("Filter Wheel Settings"=w201:T45)  [unwired: 9 in, 1 out]
            n138 = Unbundle By Name(w201) -> ("Filters"=w195:T46[])  [unwired: 1 out]
            n139 = for {
              N: 4 -> [_]
              tunnel: w195 -> [w214] mode=indexing
              tunnel: w194 -> [w213] mode=indexing
              tunnel: w187 -> [w211] mode=indexing
              w210 = TRUE ("Visible")
              n140 = Unbundle By Name(w214) -> ("Names"=w212:string[], "Wheel Name"=w209:string)
              n141 = property class="LstBox (strict)"(reference=w213, "Item Names"=w212, "Visible"=w210, "Caption.Text"=w209) -> ()  [unwired: 1 in, 2 out]
              n142 = property class="Bool"(reference=w211, "Visible"=w210) -> ()  [unwired: 1 in, 2 out]
            }
          }
          frame "save script" {
            n143 = Unbundle By Name(w230) -> ("Settings.Script"=w218:string, "Script"=w231:T20[], "Settings.Script Path"=w215:path)
            n144 = Bundle By Name(cluster=T27 {"Name"="", "Script"=[]} ("Script"), "Name"=w218, "Script"=w231) -> (w232:T27)
            n145 = Obtain Queue(name (unnamed)="Script Queue", element data type=T29 {"Cmd"="", "Parameters"=variant}) -> (queue out=w227:refnum<queue>)  [unwired: 3 in, 2 out]
            n146 = call "CC Rd Wr Script.vi"("Script Path"=w215, "Action"=CC_Rd_Wr_Script_Action."Write", "Script"=w232) -> ("error out"=w220:errorcluster, "Script List"=w219:string[])  [unwired: 3 in, 4 out]
            n147 = Bundle By Name(cluster=T29 {"Cmd"="", "Parameters"=variant} ("element"), "Cmd"="set script", "Parameters"=w218) -> (w223:T29)
            n148 = Search 1D Array(1D array=w219, element=w218) -> (index of element=w217:i32)  [unwired: 1 in]
            n149 = property on="Script Name" class="Ring (strict)"(error in=w220, "Strings []"=w219, "Value"=w217) -> (error out=w224:errorcluster)  [unwired: 1 in, 1 out]
            n150 = Enqueue Element(queue=w227, element=w223, error in (no error)=w224) -> (queue out=w221:refnum<queue>, error out=w222:errorcluster)  [unwired: 1 in, 1 out]
            n151 = Release Queue(queue=w221, error in (no error)=w222) -> ()  [unwired: 1 in, 3 out]
          }
          frame "delete script" {
            n152 = Unbundle By Name(w235) -> ("Settings.Script Path"=w234:path)
            n153 = property on="Script Name" class="Ring (strict)"() -> ("Strings []"=w243:string[], "Value"=w240:u16)  [unwired: 2 in, 2 out]
            n154 = Index Array(array=w243, index=w240) -> (element=w241:string)
            n155 = Bundle By Name(cluster=T27 {"Name"="", "Script"=[]} ("Script"), "Name"=w241) -> (w245:T27)
            n156 = call "CC Rd Wr Script.vi"("Script Path"=w234, "Action"=CC_Rd_Wr_Script_Action."Delete", "Script"=w245) -> ("error out"=w244:errorcluster, "Script List"=w237:string[])  [unwired: 3 in, 4 out]
            n157 = Array Size(array=w237) -> (size(s)=w236:i32)
            n158 = In Range and Coerce(upper limit=w236, x=w240, lower limit=u16 0) -> (coerced(x)=w238:i32)  [unwired: 1 out]
            n159 = property on="Script Name" class="Ring (strict)"(error in=w244, "Strings []"=w237, "Val(Sgnl)"=w238) -> ()  [unwired: 1 in, 2 out]
          }
          frame "show script" {
            n160 = Unbundle By Name(w250) -> ("Script"=w249:T20[])
            n161 = call "CC Script to Table.vi"("Line Numbers?"=TRUE, "Script"=w249) -> ("table"=w248:string[][])  [unwired: 8 in, 1 out]
            n162 = property on="Script" class="MCListbox (strict)"("ItemNames"=w248) -> ()  [unwired: 2 in, 2 out]
          }
          frame "update script" {
            n163 = Unbundle By Name(w255) -> ("state"=w254:refnum<user-event>)
            n164 = Generate User Event(user event=w254, event data cluster="show script" ("event data")) -> (user event out=w253:refnum<user-event>)  [unwired: 2 in, 1 out]
            n165 = Generate User Event(user event=w253, event data cluster="save script" ("event data")) -> ()  [unwired: 2 in, 2 out]
          }
          frame "run test" {
            n166 = Unbundle By Name(w258) -> ("test"=w257:T20[])
            n167 = Index Array(array=w257) -> (element=w256:T20)  [unwired: 1 in]
            n168 = call "CC Script Execute Step.vi"("Script Step"=w256) -> ()  [unwired: 10 in, 1 out]
          }
        }
      }
      event "Add/Replace": Value Change {
        n169 = event-data() -> ()  [unwired: 1 in, 1 out]
        n170 = case shown="\"Integer\"" "Type" {
          tunnel: "Value" -> [w273 w276 w279]
          tunnel: [w273 w274 w277] -> w260
          frame "String", Default {
          }
          frame "Integer" {
            n171 = Decimal String To Number(string=w276) -> (number=w275:i32)  [unwired: 2 in, 1 out]
            n172 = Number To Decimal String(number=w275) -> (decimal integer string=w274:string)  [unwired: 1 in]
          }
          frame "Float" {
            n173 = Fract/Exp String To Number(string=w279) -> (number=w278:dbl)  [unwired: 3 in, 1 out]
            n174 = Number To Fractional String(number=w278) -> (F-format string=w277:string)  [unwired: 3 in]
          }
        }
        n175 = Unbundle By Name(w271) -> ("state"=w264:refnum<user-event>, "Hdr Map"=w267:map{string, T25})
        n176 = Bundle By Name(cluster=T25 {"Field Name"="", "Type"=enum."String", "Value"="", "Comment"="", "Units"=""} ("FITS Hdr Row"), "Field Name"="Header Field", "Type"="Type", "Value"=w260, "Comment"="Comment", "Units"="Units") -> (w266:T25)
        n177 = Insert Into Map(map in=w267, key="Header Field", value=w266) -> (map out=w265:map{string, T25})  [unwired: 2 out]
        n178 = Generate User Event(user event=w264, event data cluster="show fits header" ("event data")) -> ()  [unwired: 2 in, 2 out]
        n179 = Bundle By Name(cluster=w271, "Hdr Map"=w265) -> (w272:T26)
      }
      event "Header Field": Value Change {
        n180 = event-data() -> ("CtlRef"=w282:refnum<vi>, "NewVal"=w281:string)  [unwired: 1 in]
        n181 = call "FITS Filter Name.vi"("Hdr Name"=w281) -> ("Filtered Name"=w280:string)  [unwired: 9 in, 1 out]
        n182 = property class="CmbBox"(reference=w282, "Value"=w280) -> ()  [unwired: 1 in, 2 out]
      }
      event "FITS Header": Shortcut Menu Activation? {
        n183 = event-data() -> ()  [unwired: 1 in, 7 out]
        n184 = event-data("Discard?"=FALSE) -> ()  [unwired: 1 in, 1 out]
      }
      event "FITS Header": Shortcut Menu Selection (User) {
        n185 = event-data() -> ("ItemTag"=w294:string, "CtlRef"=w296:refnum<vi>, "Coords"=w295:T48)  [unwired: 1 in, 5 out]
        n186 = Unbundle By Name(w288) -> ("state"=w287:refnum<user-event>, "Hdr Map"=w291:map{string, T25})
        n187 = invoke class="MCListbox (strict)" method="Point To Row Column"(reference=w296, "Point"=w295) -> (reference out=w292:refnum<vi>, "CellPosition"=w293:T49)  [unwired: 5 in, 5 out]
        n188 = Generate User Event(user event=w287, event data cluster="show fits header" ("event data")) -> ()  [unwired: 2 in, 2 out]
        n189 = case shown="\"False\", Default" w294 {
          tunnel: w293 -> [_ w305]
          tunnel: w292 -> [_ w304]
          tunnel: w291 -> [w297 w300]
          tunnel: [w297 w298] -> w290
          frame "False", Default {
          }
          frame "Delete Item" {
            n190 = property class="MCListbox (strict)"(reference=w304) -> ("ItemNames"=w303:string[][])  [unwired: 1 in, 2 out]
            n191 = Unbundle By Name(w305) -> ("Row"=w302:i32)
            n192 = Index Array(array=w303, index (row)=w302, index (col)=0 ("disabled index (col)")) -> (element=w299:string)
            n193 = Remove From Map(10:w299, 11:w300) -> (3:w298:map{string, T25})  [unwired: 2 out]
          }
        }
        n194 = Bundle By Name(cluster=w288, "Hdr Map"=w290) -> (w289:T26)
      }
      event "FITS Header": Value Change {
        n195 = event-data() -> ("CtlRef"=w314:refnum<vi>, "NewVal"=w312:i32)  [unwired: 1 in]
        n196 = property class="MCListbox (strict)"(reference=w314) -> ("ItemNames"=w313:string[][])  [unwired: 1 in, 2 out]
        n197 = Unbundle By Name(w310) -> ("Hdr Map"=w309:map{string, T25})
        n198 = Index Array(array=w313, index (row)=w312, index (col)=0 ("disabled index (col)")) -> (element=w308:string)
        n199 = Look In Map(map=w309, key=w308) -> (key not found?=w307:bool, value=w306:T25)  [unwired: 1 in]
        n200 = case shown="False" w307 {
          tunnel: w306 -> [w320 _]
          frame False {
            n201 = Unbundle By Name(w320) -> ("Field Name"=w319:string, "Type"=w318:T2, "Value"=w317:string, "Comment"=w316:string, "Units"=w315:string)
            n202 = property on="Header Field" class="CmbBox"("Value"=w319) -> ()  [unwired: 2 in, 2 out]
            n203 = property on="Type" class="Enum (strict)"("Value"=w318) -> ()  [unwired: 2 in, 2 out]
            n204 = property on="Value" class="Str"("Value"=w317) -> ()  [unwired: 2 in, 2 out]
            n205 = property on="Units" class="Str"("Value"=w315) -> ()  [unwired: 2 in, 2 out]
            n206 = property on="Comment" class="Str"("Value"=w316) -> ()  [unwired: 2 in, 2 out]
          }
          frame True {
          }
        }
      }
      event "Open Button": Value Change {
        n207 = event-data() -> ()  [unwired: 1 in, 6 out]
        n208 = call "Rd Wr detector settings json.vi"("Detector Name"="PRIME") -> ("Detector Config"=w322:T40)  [unwired: 9 in, 1 out]
        n209 = Unbundle By Name(w322) -> ("FITS hdr template0"=w321:path)
        n210 = call <vilib>:"Show in File System.vi"("file or directory path"=w321) -> ()  [unwired: 10 in, 1 out]
      }
      event "Save Header": Value Change {
        n211 = event-data() -> ()  [unwired: 1 in, 6 out]
        n212 = call "Rd Wr detector settings json.vi"("Detector Name"="PRIME") -> ("Detector Config"=w330:T40)  [unwired: 9 in, 1 out]
        n213 = Unbundle By Name(w328) -> ("Hdr Map"=w327:map{string, T25})
        n214 = Unbundle By Name(w330) -> ("FITS hdr template0"=w329:path)
        n215 = for {
          tunnel: w327 -> [w333] mode=indexing
          tunnel: [w332] -> w326 mode=indexing
          n216 = Unbundle(w333) -> (w332:T25)  [unwired: 1 out]
        }
        n217 = call "Rd Wr FITS Header JSON.vi"("FITS Template"=w329, "Write? (F:Read)"=TRUE, "FITS Hdr Rows"=w326) -> ()  [unwired: 7 in, 2 out]
      }
      event "Script Path": Value Change {
        n218 = event-data() -> ()  [unwired: 1 in, 6 out]
        n219 = Unbundle By Name(w339) -> ("state"=w338:refnum<user-event>)
        n220 = Generate User Event(user event=w338, event data cluster="init" ("event data")) -> ()  [unwired: 2 in, 2 out]
        n221 = Bundle By Name(cluster=w339, "Settings.Script Path"="Script Path") -> (w336:T26)
        n222 = Unbundle By Name(w336) -> ("Settings"=w335:T22)
        n223 = call "Rd Wr Script Defaults.vi"("Write? (F:Read)"=TRUE, "Script Settings"=w335) -> ()  [unwired: 8 in, 2 out]
      }
      event "Telescope Focus.Focus Home": Value Change {
        n224 = event-data() -> ()  [unwired: 1 in, 6 out]
        n225 = Unbundle By Name(w341) -> ("Script"=w347:T20[], "state"=w344:refnum<user-event>)
        n226 = Generate User Event(user event=w344, event data cluster="update script" ("event data")) -> ()  [unwired: 2 in, 2 out]
        n227 = Bundle By Name(cluster=T20 {"Action"=enum."Acquire Images", "Data"=variant}, "Action"=CC_enum_Script_Action."Telescope Home") -> (w346:T20)
        n228 = Build Array (concatenate)(w347, w346) -> (w345:T20[])
        n229 = Bundle By Name(cluster=w341, "Script"=w345) -> (w342:T26)
      }
      event "Telescope Focus.Move Focus": Value Change {
        # "Telescope Focus"
        n230 = event-data() -> ()  [unwired: 1 in, 6 out]
        n231 = Unbundle By Name(w352) -> ("Script"=w358:T20[], "state"=w355:refnum<user-event>)
        n232 = Unbundle By Name("Telescope Focus") -> ("Position"=w350:dbl)
        n233 = Generate User Event(user event=w355, event data cluster="update script" ("event data")) -> ()  [unwired: 2 in, 2 out]
        n234 = Bundle By Name(cluster=T20 {"Action"=enum."Acquire Images", "Data"=variant}, "Action"=CC_enum_Script_Action."Telescope Move", "Data"=w350) -> (w357:T20)
        n235 = Build Array (concatenate)(w358, w357) -> (w356:T20[])
        n236 = Bundle By Name(cluster=w352, "Script"=w356) -> (w353:T26)
      }
      event "Move Telescope": Value Change {
        n237 = event-data() -> ()  [unwired: 1 in, 6 out]
        n238 = Unbundle By Name(w365) -> ("Script"=w371:T20[], "state"=w368:refnum<user-event>)
        n239 = Unbundle By Name("RA and DEC String 2") -> ("RA"=w363:string, "DEC"=w362:string)
        n240 = call "Telescope Convert HHMMSS to RA and DEC Angle.vi"("Dec String"=w362, "RA String"=w363) -> ("RA and DEC"=w361:T15)  [unwired: 7 in, 2 out]
        n241 = Generate User Event(user event=w368, event data cluster="update script" ("event data")) -> ()  [unwired: 2 in, 2 out]
        n242 = Bundle By Name(cluster=T20 {"Action"=enum."Acquire Images", "Data"=variant}, "Action"=CC_enum_Script_Action."Telescope RA DEC", "Data"=w361) -> (w370:T20)
        n243 = Build Array (concatenate)(w371, w370) -> (w369:T20[])
        n244 = Bundle By Name(cluster=w365, "Script"=w369) -> (w366:T26)
      }
      event "Relative", "Absolute": Value Change {
        n245 = event-data() -> ()  [unwired: 1 in, 6 out]
        n246 = Unbundle By Name(w386) -> ("state"=w388:refnum<user-event>, "Script"=w389:T20[])
        n247 = Bundle By Name(cluster=T30 {"Motor"=0, "Position"=0} ("Cluster"), "Motor"="Select Motor (0:n-1)", "Position"="Steps") -> (w378:T30)
        n248 = Select(t=CC_enum_Script_Action."Focus Move Absolute" ("Action"), s="Absolute", f=CC_enum_Script_Action."Focus Move Relative" ("Action")) -> (s? t:f=w376:T21)
        n249 = Bundle By Name(cluster=T20 {"Action"=enum."Acquire Images", "Data"=variant}, "Action"=w376, "Data"=w378) -> (w384:T20)
        n250 = Generate User Event(user event=w388, event data cluster="update script" ("event data")) -> ()  [unwired: 2 in, 2 out]
        n251 = Build Array (concatenate)(w389, w384) -> (w383:T20[])
        n252 = Bundle By Name(cluster=w386, "Script"=w383) -> (w387:T26)
      }
      event "Add Outlet Cmd": Value Change {
        n253 = event-data() -> ()  [unwired: 1 in, 6 out]
        n254 = Bundle By Name(cluster=T31 {"Outlet Idx"=0, "State"=FALSE}, "Outlet Idx"="Outlet Index (0 based)", "State"="Outlet State") -> (w398:T31)
        n255 = Unbundle By Name(w392) -> ("state"=w395:refnum<user-event>, "Script"=w396:T20[])
        n256 = Bundle By Name(cluster=T20 {"Action"=enum."Acquire Images", "Data"=variant}, "Action"=CC_enum_Script_Action."Outlet", "Data"=w398) -> (w391:T20)
        n257 = Generate User Event(user event=w395, event data cluster="update script" ("event data")) -> ()  [unwired: 2 in, 2 out]
        n258 = Build Array (concatenate)(w396, w391) -> (w394:T20[])
        n259 = Bundle By Name(cluster=w392, "Script"=w394) -> (w390:T26)
      }
      event "Home Focus": Value Change {
        n260 = event-data() -> ()  [unwired: 1 in, 6 out]
        n261 = local read "Select Motor (0:n-1)"() -> (w405:i32)
        n262 = Unbundle By Name(w403) -> ("state"=w411:refnum<user-event>, "Script"=w412:T20[])
        n263 = Bundle By Name(cluster=T20 {"Action"=enum."Acquire Images", "Data"=variant}, "Action"=CC_enum_Script_Action."Focus Set Home", "Data"=w405) -> (w409:T20)
        n264 = Generate User Event(user event=w411, event data cluster="update script" ("event data")) -> ()  [unwired: 2 in, 2 out]
        n265 = Build Array (concatenate)(w412, w409) -> (w408:T20[])
        n266 = Bundle By Name(cluster=w403, "Script"=w408) -> (w404:T26)
      }
      event "Objects": Value Change {
        n267 = event-data() -> ("CtlRef"=w421:refnum<vi>, "NewVal"=w419:i32)  [unwired: 1 in]
        n268 = property class="MCListbox (strict)"(reference=w421) -> ("ItemNames"=w420:string[][])  [unwired: 1 in, 2 out]
        n269 = Unbundle By Name(w415) -> ("state"=w414:refnum<user-event>)
        n270 = Generate User Event(user event=w414, event data cluster="show object" ("event data")) -> ()  [unwired: 2 in, 2 out]
        n271 = Index Array(array=w420, index (row)=w419, index (col)=0 ("disabled index (col)")) -> (element=w417:string)
        n272 = Bundle By Name(cluster=w415, "curr object"=w417) -> (w416:T26)
      }
      event "Obj Add/Replace": Value Change {
        n273 = event-data() -> ()  [unwired: 1 in, 1 out]
        n274 = call "CC RA and DEC to decimal.vi"("RA and DEC String"="RA and DEC String") -> ("error out"=w422:errorcluster, "RA and DEC"=w424:T15)  [unwired: 9 in]
        n275 = case shown="No Error" w422 {
          tunnel: [w430 w442] -> w426
          tunnel: w425 -> [w429 w442]
          tunnel: w424 -> [w428 _]
          frame No Error {
            n276 = Unbundle By Name(w429) -> ("state"=w433:refnum<user-event>, "Object Map"=w440:map{string, T14})
            n277 = Unbundle By Name("Object Name") -> ("Name"=w439:string)
            n278 = Bundle By Name(cluster=T14 {"Object"={"Name"=""}, "Sidereal Rate"={"dRA"=0.0, "dDEC"=0.0}, "RA and DEC"={"RA"=0.0, "DEC"=0.0}, "Proper Motion"={"muRA"=0.0, "muDEC"=0.0, "Epoch"=0.0}, "Offsets"={"RA"=0.0, "DEC"=0.0, "ROT"=0.0}, "Equinox"={"Equinox Year"=2000, "Equinox Prefix"="J"}, "Parallax"={"Parallax"=0.0, "rv kps"=0.0}, "Rotator"={"Frame"="", "PA"=0.0}, "Frame"=enum."FK5", "Frac Rate"=1.0, "Wavelength"=0.5} ("value"), "Object"="Object Name", "Sidereal Rate"="Sidereal Rate", "RA and DEC"=w428, "Proper Motion"="Proper Motion", "Offsets"="Offsets") -> (w434:T14)
            n279 = Generate User Event(user event=w433, event data cluster="show object list" ("event data")) -> ()  [unwired: 2 in, 2 out]
            n280 = Insert Into Map(map in=w440, key=w439, value=w434) -> (map out=w431:map{string, T14})  [unwired: 2 out]
            n281 = Bundle By Name(cluster=w429, "Object Map"=w431) -> (w430:T26)
          }
          frame Error {
            n282 = One Button Dialog(message="RA and/or DEC invalid format. \nRA format: HH:MM:SS.nnn\nDEC format: DEG:arcmin:arcsec.nn") -> ()  [unwired: 1 in, 1 out]
          }
        }
      }
      event "Obj Remove": Value Change {
        n283 = event-data() -> ()  [unwired: 1 in, 1 out]
        n284 = Unbundle By Name(w445) -> ("Object Map"=w455:map{string, T14}, "state"=w443:refnum<user-event>)
        n285 = property on="Objects" class="MCListbox (strict)"() -> ("ItemNames"=w457:string[][], "Value"=w450:i32)  [unwired: 2 in, 2 out]
        n286 = Generate User Event(user event=w443, event data cluster="show object list" ("event data")) -> (error out=w444:errorcluster)  [unwired: 2 in, 1 out]
        n287 = Index Array(array=w457, index (row)=w450, index (col)=0 ("disabled index (col)")) -> (element=w454:string)
        n288 = Remove From Map(10:w454, 11:w455) -> (3:w452:map{string, T14})  [unwired: 2 out]
        n289 = Collection Size(1:w452) -> (0:w449:i32)
        n290 = Bundle By Name(cluster=w445, "Object Map"=w452) -> (w446:T26)
        n291 = Greater Or Equal?(x=w449, y=w450) -> (x >= y?=w451:bool)
        n292 = Decrement(x=w449) -> (x-1=w448:i32)
        n293 = Select(t=w448, s=w451, f=w450) -> (s? t:f=w447:i32)
        n294 = property on="Objects" class="MCListbox (strict)"(error in=w444, "Val(Sgnl)"=w447) -> ()  [unwired: 1 in, 2 out]
      }
      event "Obj Add to Script": Value Change {
        n295 = event-data() -> ()  [unwired: 1 in, 6 out]
        n296 = Unbundle By Name(w460) -> ("state"=w458:refnum<user-event>, "Script"=w461:T20[], "Object Map"=w465:map{string, T14})
        n297 = property on="Objects" class="MCListbox (strict)"() -> ("ItemNames"=w468:string[][], "Value"=w467:i32)  [unwired: 2 in, 2 out]
        n298 = Index Array(array=w468, index (row)=w467, index (col)=0 ("disabled index (col)")) -> (element=w464:string)
        n299 = Look In Map(map=w465, key=w464) -> (key not found?=w463:bool, value=w462:T14)  [unwired: 1 in]
        n300 = case shown="False" w463 {
          tunnel: w462 -> [w476 _]
          tunnel: w461 -> [w474 _]
          tunnel: w460 -> [w473 w479]
          tunnel: [w471 w479] -> w459
          tunnel: w458 -> [w470 _]
          frame False {
            n301 = Generate User Event(user event=w470, event data cluster="update script" ("event data")) -> ()  [unwired: 2 in, 2 out]
            n302 = Bundle By Name(cluster=T20 {"Action"=enum."Acquire Images", "Data"=variant}, "Action"=CC_enum_Script_Action."Define Object", "Data"=w476) -> (w475:T20)
            n303 = Build Array (concatenate)(w474, w475) -> (w472:T20[])
            n304 = Bundle By Name(cluster=w473, "Script"=w472) -> (w471:T26)
          }
          frame True {
            n305 = One Button Dialog(message="Add Object to List before adding to script.") -> ()  [unwired: 1 in, 1 out]
          }
        }
      }
      event "Exp Add to Script": Value Change {
        n306 = event-data() -> ()  [unwired: 1 in, 6 out]
        n307 = Unbundle By Name(w483) -> ("state"=w481:refnum<user-event>, "Script"=w484:T20[], "Exp Map"=w488:map{string, T6})
        n308 = property on="Exposures" class="MCListbox (strict)"() -> ("ItemNames"=w491:string[][], "Value"=w490:i32)  [unwired: 2 in, 2 out]
        n309 = Index Array(array=w491, index (row)=w490, index (col)=0 ("disabled index (col)")) -> (element=w487:string)
        n310 = Look In Map(map=w488, key=w487) -> (key not found?=w486:bool, value=w485:T6)  [unwired: 1 in]
        n311 = case shown="False" w486 {
          tunnel: w485 -> [w499 _]
          tunnel: w484 -> [w497 _]
          tunnel: w483 -> [w496 w502]
          tunnel: [w494 w502] -> w482
          tunnel: w481 -> [w493 _]
          frame False {
            n312 = Generate User Event(user event=w493, event data cluster="update script" ("event data")) -> ()  [unwired: 2 in, 2 out]
            n313 = Bundle By Name(cluster=T20 {"Action"=enum."Acquire Images", "Data"=variant}, "Action"=CC_enum_Script_Action."Define Exposure", "Data"=w499) -> (w498:T20)
            n314 = Build Array (concatenate)(w497, w498) -> (w495:T20[])
            n315 = Bundle By Name(cluster=w496, "Script"=w495) -> (w494:T26)
          }
          frame True {
            n316 = One Button Dialog(message="Add Object to List before adding to script.") -> ()  [unwired: 1 in, 1 out]
          }
        }
      }
      event "Dither Add to Script": Value Change {
        n317 = event-data() -> ()  [unwired: 1 in, 1 out]
        n318 = Unbundle By Name(w508) -> ("state"=w506:refnum<user-event>, "Script"=w509:T20[], "Dither Map"=w511:map{string, T23})
        n319 = property on="Dithering" class="MCListbox (strict)"() -> ("ItemNames"=w514:string[][], "Value"=w513:i32)  [unwired: 2 in, 2 out]
        n320 = Index Array(array=w514, index (row)=w513, index (col)=1 ("disabled index (col)")) -> (element=w504:string)
        n321 = Look In Map(map=w511, key=w504) -> (key not found?=w510:bool, value=w505:T23)  [unwired: 1 in]
        n322 = case shown="False" w510 {
          tunnel: w509 -> [w525 _]
          tunnel: w508 -> [w524 w537]
          tunnel: [w522 w537] -> w507
          tunnel: w506 -> [w521 _]
          tunnel: w505 -> [w519 _]
          tunnel: w504 -> [w515 _]
          frame False {
            n323 = Unbundle By Name(w519) -> ("Dithering Type"=w518:T24, "Random Dither"=w516:T8, "Dithering Offsets"=w517:T9)
            n324 = Generate User Event(user event=w521, event data cluster="update script" ("event data")) -> ()  [unwired: 2 in, 2 out]
            n325 = case shown="\"Random\", Default" w518 {
              tunnel: [w530 w535] -> w526
              tunnel: w517 -> [_ w534]
              tunnel: w516 -> [w528 _]
              tunnel: w515 -> [w527 w533]
              frame "Random", Default {
                n326 = Bundle By Name(cluster=w528, "Name"=w527) -> (w529:T8)
                n327 = Bundle By Name(cluster=T20 {"Action"=enum."Define Random Dither", "Data"=variant}, "Data"=w529) -> (w530:T20)
              }
              frame "Offsets" {
                n328 = Bundle By Name(cluster=w534, "Name"=w533) -> (w532:T9)
                n329 = Bundle By Name(cluster=T20 {"Action"=enum."Define Dithering", "Data"=variant}, "Data"=w532) -> (w535:T20)
              }
            }
            n330 = Build Array (concatenate)(w525, w526) -> (w523:T20[])
            n331 = Bundle By Name(cluster=w524, "Script"=w523) -> (w522:T26)
          }
          frame True {
            n332 = One Button Dialog(message="Add Object to List before adding to script.") -> ()  [unwired: 1 in, 1 out]
          }
        }
      }
      event "Exposures": Value Change {
        n333 = event-data() -> ("CtlRef"=w542:refnum<vi>, "NewVal"=w541:i32)  [unwired: 1 in]
        n334 = property class="MCListbox (strict)"(reference=w542) -> ("ItemNames"=w547:string[][])  [unwired: 1 in, 2 out]
        n335 = Unbundle By Name(w539) -> ("state"=w544:refnum<user-event>)
        n336 = Generate User Event(user event=w544, event data cluster="show exp" ("event data")) -> ()  [unwired: 2 in, 2 out]
        n337 = Index Array(array=w547, index (row)=w541, index (col)=0 ("disabled index (col)")) -> (element=w545:string)
        n338 = Bundle By Name(cluster=w539, "curr object"=w545) -> (w540:T26)
      }
      event "Exp Add/Replace": Value Change {
        n339 = event-data() -> ()  [unwired: 1 in, 6 out]
        n340 = Unbundle By Name(w550) -> ("state"=w549:refnum<user-event>, "Exp Map"=w555:map{string, T6})
        n341 = Unbundle By Name("Exposure") -> ("Name"=w554:string)
        n342 = Insert Into Map(map in=w555, key=w554, value="Exposure") -> (map out=w552:map{string, T6})  [unwired: 2 out]
        n343 = Generate User Event(user event=w549, event data cluster="show exp list" ("event data")) -> ()  [unwired: 2 in, 2 out]
        n344 = Bundle By Name(cluster=w550, "Exp Map"=w552) -> (w551:T26)
      }
      event "Exp Remove": Value Change {
        n345 = event-data() -> ()  [unwired: 1 in, 6 out]
        n346 = Unbundle By Name(w556) -> ("Exp Map"=w568:map{string, T6}, "state"=w558:refnum<user-event>)
        n347 = property on="Exposures" class="MCListbox (strict)"() -> ("ItemNames"=w570:string[][], "Value"=w563:i32)  [unwired: 2 in, 2 out]
        n348 = Generate User Event(user event=w558, event data cluster="show exp list" ("event data")) -> (error out=w559:errorcluster)  [unwired: 2 in, 1 out]
        n349 = Index Array(array=w570, index (row)=w563, index (col)=0 ("disabled index (col)")) -> (element=w567:string)
        n350 = Remove From Map(10:w567, 11:w568) -> (3:w565:map{string, T6})  [unwired: 2 out]
        n351 = Collection Size(1:w565) -> (0:w562:i32)
        n352 = Bundle By Name(cluster=w556, "Exp Map"=w565) -> (w557:T26)
        n353 = Greater Or Equal?(x=w562, y=w563) -> (x >= y?=w564:bool)
        n354 = Decrement(x=w562) -> (x-1=w561:i32)
        n355 = Select(t=w561, s=w564, f=w563) -> (s? t:f=w560:i32)
        n356 = property on="Exposures" class="MCListbox (strict)"(error in=w559, "Val(Sgnl)"=w560) -> ()  [unwired: 1 in, 2 out]
      }
      event "Dithering": Value Change {
        n357 = event-data() -> ("CtlRef"=w574:refnum<vi>, "NewVal"=w573:i32)  [unwired: 1 in, 4 out]
        n358 = property class="MCListbox (strict)"(reference=w574) -> ("ItemNames"=w579:string[][])  [unwired: 1 in, 2 out]
        n359 = Unbundle By Name(w571) -> ("state"=w576:refnum<user-event>)
        n360 = Generate User Event(user event=w576, event data cluster="show dither" ("event data")) -> ()  [unwired: 2 in, 2 out]
        n361 = Index Array(array=w579, index (row)=w573, index (col)=1 ("disabled index (col)")) -> (element=w577:string)
        n362 = Bundle By Name(cluster=w571, "curr object"=w577) -> (w572:T26)
      }
      event "Dithering Add/Replace": Value Change {
        n363 = event-data() -> ()  [unwired: 1 in, 6 out]
        n364 = case shown="\"Offset\"" "Dither Select" {
          tunnel: [w594 w605] -> w586
          tunnel: w585 -> [w593 w604]
          tunnel: "Name" -> [w590 w602]
          tunnel: [w589 w601] -> w581
          tunnel: T23 {"Name"="", "Dithering Offsets"={"Name"="", "Dithering Offsets"={"Offsets"=[]}}, "Dithering Type"=enum."Random", "Random Dither"={"Count"=1, "Radius"=1.0, "Name"=""}} ("value") -> [w588 w599]
          frame "Random", Default {
            n365 = Unbundle By Name(w593) -> ("state"=w596:refnum<user-event>, "Dither Map"=w597:map{string, T23})
            n366 = Bundle By Name(cluster=w588, "Name"=w590, "Dithering Type"=CC_enum_Dithering_Types."Random", "Random Dither"="Random Dither") -> (w587:T23)
            n367 = Insert Into Map(map in=w597, key=w590, value=w587) -> (map out=w589:map{string, T23})  [unwired: 2 out]
            n368 = Generate User Event(user event=w596, event data cluster="show dither list" ("event data")) -> ()  [unwired: 2 in, 2 out]
            n369 = Bundle By Name(cluster=w593, "Dither Map"=w589) -> (w594:T26)
          }
          frame "Offset" {
            n370 = Unbundle By Name(w604) -> ("state"=w607:refnum<user-event>, "Dither Map"=w608:map{string, T23})
            n371 = Bundle By Name(cluster=w599, "Name"=w602, "Dithering Type"=CC_enum_Dithering_Types."Offsets", "Dithering Offsets"="Dithering Offset") -> (w598:T23)
            n372 = Generate User Event(user event=w607, event data cluster="show dither list" ("event data")) -> ()  [unwired: 2 in, 2 out]
            n373 = Insert Into Map(map in=w608, key=w602, value=w598) -> (map out=w601:map{string, T23})  [unwired: 2 out]
            n374 = Bundle By Name(cluster=w604, "Dither Map"=w601) -> (w605:T26)
          }
        }
        n375 = call "CC Rd Wr Dither Map.vi"("Write? (F:Read)"=TRUE, "Dither Map"=w581) -> ()  [unwired: 8 in, 2 out]
      }
      event "Dithering Remove": Value Change {
        n376 = event-data() -> ()  [unwired: 1 in, 6 out]
        n377 = Unbundle By Name(w622) -> ("Dither Map"=w621:map{string, T23}, "state"=w624:refnum<user-event>)
        n378 = property on="Dither Select" class="TabCtl (strict)" props=["Value"]() -> ()  [unwired: 2 in, 3 out]
        n379 = property on="Dithering" class="MCListbox (strict)"() -> ("ItemNames"=w620:string[][], "Value"=w615:i32)  [unwired: 2 in, 2 out]
        n380 = Index Array(array=w620, index (row)=w615, index (col)=1 ("disabled index (col)")) -> (element=w618:string)
        n381 = Generate User Event(user event=w624, event data cluster="show dither list" ("event data")) -> (error out=w611:errorcluster)  [unwired: 2 in, 1 out]
        n382 = Remove From Map(10:w618, 11:w621) -> (3:w609:map{string, T23})  [unwired: 2 out]
        n383 = Collection Size(1:w609) -> (0:w614:i32)
        n384 = Greater Or Equal?(x=w614, y=w615) -> (x >= y?=w616:bool)
        n385 = Bundle By Name(cluster=w622, "Dither Map"=w609) -> (w623:T26)
        n386 = Decrement(x=w614) -> (x-1=w613:i32)
        n387 = Select(t=w613, s=w616, f=w615) -> (s? t:f=w612:i32)
        n388 = call "CC Rd Wr Dither Map.vi"("Write? (F:Read)"=TRUE, "Dither Map"=w609) -> ()  [unwired: 8 in, 2 out]
        n389 = property on="Dithering" class="MCListbox (strict)"(error in=w611, "Val(Sgnl)"=w612) -> ()  [unwired: 1 in, 2 out]
      }
      event "Add FW 1", "Add FW 2", "Add FW 3", "Add FW 4": Value Change {
        # "MoveFilterWheel\nSyntax:\nMoveFilterWheel Wheel1:n,Wheel2:n\nParameter\tUnits\tPurpose\nWheel1\t\tPosition of Wheel one (integer)\nWheel2\t\tPosition of Wheel two (integer)"
        n390 = event-data() -> ("CtlRef"=w642:refnum<vi>)  [unwired: 1 in, 2 out]
        n391 = property class="Bool"(reference=w642) -> ("Label.Text"=w641:string)  [unwired: 1 in, 2 out]
        n392 = Unbundle By Name(w628) -> ("state"=w630:refnum<user-event>, "Script"=w629:T20[])
        n393 = Build Array("Filter Wheel 1", "Filter Wheel 2", "Filter Wheel 3", "Filter Wheel 4") -> (w634:i32[])
        n394 = Match Pattern(string=w641, regular expression="Add FW ") -> (after substring=w639:string)  [unwired: 1 in, 3 out]
        n395 = Decimal String To Number(string=w639) -> (number=w633:i32)  [unwired: 2 in, 1 out]
        n396 = Decrement(x=w633) -> (x-1=w625:i32)
        n397 = Index Array(array=w634, index=w625) -> (element=w632:i32)
        n398 = Bundle By Name(cluster=T32 {"Wheel"=0, "Filter"=0} ("Acquire Parameters in"), "Wheel"=w625, "Filter"=w632) -> (w631:T32)
        n399 = Generate User Event(user event=w630, event data cluster="update script" ("event data")) -> ()  [unwired: 2 in, 2 out]
        n400 = Bundle By Name(cluster=T20 {"Action"=enum."Acquire Images", "Data"=variant}, "Action"=CC_enum_Script_Action."Set Filter Wheel", "Data"=w631) -> (w645:T20)
        n401 = Build Array (concatenate)(w629, w645) -> (w644:T20[])
        n402 = Bundle By Name(cluster=w628, "Script"=w644) -> (w627:T26)
      }
      event "Tab Control": Value Change {
        n403 = event-data() -> ("NewVal"=w650:T1)  [unwired: 1 in]
        n404 = case shown="\"Setup\", Default" w650 {
          tunnel: w649 -> [_ _ w679 w685]
          tunnel: "Script" -> [_ _ _ w683]
          frame "Setup", Default {
          }
          frame "Acquire" {
            w651 = refnum<vi> refnum  # ComboBox
            n405 = property on="Objects" class="MCListbox (strict)"() -> ("ItemNames"=w676:string[][], "Value"=w670:i32)  [unwired: 2 in, 2 out]
            n406 = property on="Exposures" class="MCListbox (strict)"() -> ("ItemNames"=w661:string[][], "Value"=w660:i32)  [unwired: 2 in, 2 out]
            n407 = property on="Dithering" class="MCListbox (strict)"() -> ("ItemNames"=w662:string[][], "Value"=w659:i32)  [unwired: 2 in, 2 out]
            n408 = property on="Acquire Parameters" class="Clust (strict)"() -> ("Controls[]"=w675:refnum<vi>[])  [unwired: 2 in, 2 out]
            n409 = Index Array(array=w676, index (col)=0 ("disabled index (col)")) -> (element=w671:string[])  [unwired: 1 in]
            n410 = Index Array(array=w661, index (col)=0 ("disabled index (col)")) -> (element=w667:string[])  [unwired: 1 in]
            n411 = Index Array(array=w662, index (col)=1 ("disabled index (col)")) -> (element=w664:string[])  [unwired: 1 in]
            n412 = Index Array(array=w671, index=w670) -> (element=w669:string)
            n413 = Index Array(array=w667, index=w660) -> (element=w668:string)
            n414 = Index Array(array=w675) -> (element #1=w674:refnum<vi>, element #2=w656:refnum<vi>, element #3=w653:refnum<vi>)  [unwired: 3 in]
            n415 = Index Array(array=w664, index=w659) -> (element=w663:string)
            n416 = To More Specific Class(target class=w651, reference=w674) -> (specific class reference=w673:refnum<vi>, error out=w652:errorcluster)  [unwired: 1 in]
            n417 = To More Specific Class(target class=w651, reference=w656) -> (specific class reference=w658:refnum<vi>, error out=w657:errorcluster)  [unwired: 1 in]
            n418 = To More Specific Class(target class=w651, reference=w653) -> (specific class reference=w655:refnum<vi>, error out=w654:errorcluster)  [unwired: 1 in]
            n419 = property class="CmbBox"(reference=w673, error in=w652, "Strings[]"=w671, "Value"=w669) -> ()  [unwired: 2 out]
            n420 = property class="CmbBox"(reference=w658, error in=w657, "Strings[]"=w667, "Value"=w668) -> ()  [unwired: 2 out]
            n421 = property class="CmbBox"(reference=w655, error in=w654, "Strings[]"=w664, "Value"=w663) -> ()  [unwired: 2 out]
          }
          frame "Text" {
            n422 = Unbundle By Name(w679) -> ("Script"=w678:T20[])
            n423 = call "CC Generate Script Text.vi"("Script"=w678) -> ("Script String"=→"Script As Text":string)  [unwired: 9 in, 1 out]
          }
          frame "Test" {
            n424 = Unbundle By Name(w685) -> ("Script"=w684:T20[])
            n425 = Index Array(array=w684, index=w683) -> (element=w682:T20)
            n426 = Build Array(w682) -> (w681:T20[])
            n427 = call "CC Generate Script Text.vi"("Script"=w681) -> ("Script String"=w680:string)  [unwired: 9 in, 1 out]
            n428 = property on="Script Line" class="Str"("Value"=w680) -> ()  [unwired: 2 in, 2 out]
          }
        }
      }
      event "Add Image Acq": Value Change {
        n429 = event-data() -> ()  [unwired: 1 in, 6 out]
        n430 = Unbundle By Name(w688) -> ("Script"=w692:T20[], "state"=w687:refnum<user-event>)
        n431 = Generate User Event(user event=w687, event data cluster="update script" ("event data")) -> ()  [unwired: 2 in, 2 out]
        n432 = Bundle By Name(cluster=T20 {"Action"=enum."Acquire Images", "Data"=variant}, "Action"=CC_enum_Script_Action."Acquire Images", "Data"="Acquire Parameters") -> (w691:T20)
        n433 = Build Array (concatenate)(w692, w691) -> (w690:T20[])
        n434 = Bundle By Name(cluster=w688, "Script"=w690) -> (w689:T26)
      }
      event "New Button": Value Change {
        n435 = event-data() -> ()  [unwired: 1 in, 6 out]
        n436 = Unbundle By Name(w699) -> ("state"=w698:refnum<user-event>)
        n437 = call "Script Name2"() -> ("Script Name"=w697:string, "OK"=w696:bool)  [unwired: 17 in, 1 out]
        n438 = case shown="True" w696 {
          tunnel: [w701 w709] -> w700
          tunnel: w699 -> [w701 w708]
          tunnel: w698 -> [_ w707]
          tunnel: w697 -> [_ w705]
          frame False {
          }
          frame True {
            n439 = property on="Script Name" class="Ring (strict)"() -> ("Strings []"=w703:string[])  [unwired: 2 in, 2 out]
            n440 = Generate User Event(user event=w707, event data cluster="update script" ("event data")) -> ()  [unwired: 2 in, 2 out]
            n441 = Build Array (concatenate)(w703, w705) -> (w704:string[])
            n442 = Array Size(array=w703) -> (size(s)=w702:i32)
            n443 = Bundle By Name(cluster=w708, "Settings.Script"=w705, "Script"=T20[] []) -> (w709:T26)
            n444 = property on="Script Name" class="Ring (strict)"("Strings []"=w704, "Value"=w702) -> ()  [unwired: 2 in, 2 out]
          }
        }
      }
      event "Save Script": Value Change {
        n445 = event-data() -> ()  [unwired: 1 in, 6 out]
        n446 = Unbundle By Name(w711) -> ("state"=w713:refnum<user-event>)
        n447 = Generate User Event(user event=w713, event data cluster="save script" ("event data")) -> ()  [unwired: 2 in, 2 out]
      }
      event "Save As Button": Value Change {
        n448 = event-data() -> ()  [unwired: 1 in, 6 out]
        n449 = call "Script Name"() -> ("Script Name"=w714:string, "OK"=w718:bool)  [unwired: 17 in, 1 out]
        n450 = Unbundle By Name(w716) -> ("state"=w717:refnum<user-event>)
        n451 = case shown="True" w718 {
          tunnel: w717 -> [_ w724]
          tunnel: w716 -> [w719 w720]
          tunnel: [w719 w721] -> w715
          tunnel: w714 -> [_ w722]
          frame False {
          }
          frame True {
            n452 = Bundle By Name(cluster=w720, "Settings.Script"=w722) -> (w721:T26)
            n453 = Generate User Event(user event=w724, event data cluster="save script" ("event data")) -> ()  [unwired: 2 in, 2 out]
          }
        }
      }
      event "Delete": Value Change {
        n454 = event-data() -> ()  [unwired: 1 in, 6 out]
        n455 = Unbundle By Name(w727) -> ("state"=w726:refnum<user-event>)
        n456 = Generate User Event(user event=w726, event data cluster="delete script" ("event data")) -> ()  [unwired: 2 in, 2 out]
      }
      event "Script Name": Value Change {
        n457 = event-data() -> ("NewVal"=w729:u16)  [unwired: 1 in]
        n458 = Unbundle By Name(w733) -> ("state"=w732:refnum<user-event>)
        n459 = property on="Script Name" class="Ring (strict)"() -> ("Strings []"=w730:string[])  [unwired: 2 in, 2 out]
        n460 = Generate User Event(user event=w732, event data cluster="load script" ("event data")) -> ()  [unwired: 2 in, 2 out]
        n461 = Index Array(array=w730, index=w729) -> (element=w728:string)
        n462 = Bundle By Name(cluster=w733, "Settings.Script"=w728) -> (w734:T26)
      }
      event "Script": Double Click {
        n463 = event-data() -> ("Row"=w739:i32)  [unwired: 1 in]
        n464 = Unbundle By Name(w741) -> ("Script"=w740:T20[])
        n465 = Index Array(array=w740, index=w739) -> (element=w738:T20)
        n466 = Unbundle By Name(w738) -> ("Action"=w737:T21, "Data"=w736:variant)
        n467 = case shown="\"Define Object\"" w737 {
          tunnel: [T33."Noop" ("Value (Signaling)") T33."Object" ("Value (Signaling)") T34."Exposure" ("Value (Signaling)") T33."Dithering" ("Value (Signaling)") u32 0 ("Value (Signaling)") T33."Acquire" ("Value (Signaling)") T33."Filter Wheel" ("Value (Signaling)") T36."Telescope" ("Value (Signaling)") T33."Focus" ("Value (Signaling)") T33."Focus" ("Value (Signaling)") T33."Macro" ("Value (Signaling)") T33."Pause" ("Value (Signaling)") T33."Ask" ("Value (Signaling)") T33."Dithering" ("Value (Signaling)") u32 0 ("Value (Signaling)")] -> w735
          tunnel: w736 -> [_ w754 w758 w763 _ w768 _ _ _ _ _ w778 w782 w785 _]
          frame "Noop", Default {
          }
          frame "Define Object" {
            (unwired) T50."Object" ("Value (Signaling)")
            n468 = Variant To Data(type=T14 {"Object"={"Name"=""}, "Sidereal Rate"={"dRA"=0.0, "dDEC"=0.0}, "RA and DEC"={"RA"=0.0, "DEC"=0.0}, "Proper Motion"={"muRA"=0.0, "muDEC"=0.0, "Epoch"=0.0}, "Offsets"={"RA"=0.0, "DEC"=0.0, "ROT"=0.0}, "Equinox"={"Equinox Year"=2000, "Equinox Prefix"="J"}, "Parallax"={"Parallax"=0.0, "rv kps"=0.0}, "Rotator"={"Frame"="", "PA"=0.0}, "Frame"=enum."FK5", "Frac Rate"=1.0, "Wavelength"=0.5} ("Object"), Variant=w754) -> (data=w752:T14)  [unwired: 1 in, 1 out]
            n469 = Unbundle By Name(w752) -> ("Object"=w743:cluster{"Name":string}, "Sidereal Rate"=w751:T3, "RA and DEC"=w746:T15, "Proper Motion"=w750:T4, "Offsets"=w749:T5)
            n470 = call "CC Convert RA and DEC to HHMMSS.vi"("RA and DEC"=w746) -> ("DEC String"=w745:string, "RA String"=w748:string)  [unwired: 7 in, 2 out]
            n471 = property on="Offsets" class="Clust (strict)"("Val(Sgnl)"=w749) -> ()  [unwired: 2 in, 2 out]
            n472 = property on="muRA muDEC" class="Clust (strict)"("Val(Sgnl)"=w750) -> ()  [unwired: 2 in, 2 out]
            n473 = property on="Object Name" class="Clust (strict)"("Val(Sgnl)"=w743) -> ()  [unwired: 2 in, 2 out]
            n474 = property on="Sidereal Rate" class="Clust (strict)"("Val(Sgnl)"=w751) -> ()  [unwired: 2 in, 2 out]
            n475 = Bundle("RA String"=w748, "DEC String"=w745) -> (w747:cluster{"RA String":string, "DEC String":string})  [unwired: 1 in]
            n476 = local write "RA and DEC String"(w747) -> ()
          }
          frame "Define Exposure" {
            n477 = Variant To Data(type=T6 {"Mode"=enum."CDS", "Integration Time"=1.0, "Name"="", "Images"=1} ("Exposure"), Variant=w758) -> (data=w756:T6)  [unwired: 1 in, 1 out]
            n478 = property on="Exposure" class="Clust (strict)"("Val(Sgnl)"=w756) -> ()  [unwired: 2 in, 2 out]
          }
          frame "Define Dithering" {
            n479 = Variant To Data(type=T9 {"Name"="", "Dithering Offsets"={"Offsets"=[]}} ("Dithering Offsets"), Variant=w763) -> (data=w759:T9)  [unwired: 1 in, 1 out]
            n480 = Unbundle By Name(w759) -> ("Name"=w761:string)
            n481 = property on="Dithering Offset" class="Clust (strict)"("Val(Sgnl)"=w759) -> ()  [unwired: 2 in, 2 out]
            n482 = property on="Name" class="Str"("Value"=w761) -> ()  [unwired: 2 in, 2 out]
          }
          frame "Telescope Move" {
          }
          frame "Acquire Images" {
            n483 = Variant To Data(type=T35 {"Object"="", "Exposure"="", "Dithering"=""} ("Acquire Parameters"), Variant=w768) -> (data=w766:T35)  [unwired: 1 in, 1 out]
            n484 = property on="Acquire Parameters" class="Clust (strict)"("Val(Sgnl)"=w766) -> ()  [unwired: 2 in, 2 out]
          }
          frame "Set Filter Wheel" {
          }
          frame "Telescope Home" {
          }
          frame "Focus Move Absolute" {
          }
          frame "Focus Set Home" {
          }
          frame "Macro" {
          }
          frame "Pause" {
            n485 = Variant To Data(type=T37 {"Time (s)"=0.0} ("Pause Parameters"), Variant=w778) -> (data=w776:T37)  [unwired: 1 in, 1 out]
            n486 = Unbundle By Name(w776) -> ("Time (s)"=w775:dbl)
            n487 = property on="Seconds to Pause" class="DigNum (strict)"("Val(Sgnl)"=w775) -> ()  [unwired: 2 in, 2 out]
          }
          frame "Ask User" {
            n488 = Variant To Data(type="", Variant=w782) -> (data=w780:string)  [unwired: 1 in, 1 out]
            n489 = property on="Message for User" class="Str"("Val(Sgnl)"=w780) -> ()  [unwired: 2 in, 2 out]
          }
          frame "Define Random Dither" {
            n490 = Variant To Data(type=T8 {"Count"=1, "Radius"=1.0, "Name"=""} ("Dithering Offsets"), Variant=w785) -> (data=w784:T8)  [unwired: 1 in, 1 out]
            n491 = Unbundle By Name(w784) -> ("Name"=w783:string)
            n492 = property on="Random Dither" class="Clust (strict)"("Value"=w784) -> ()  [unwired: 2 in, 2 out]
            n493 = property on="Name" class="Str"("Value"=w783) -> ()  [unwired: 2 in, 2 out]
          }
          frame "Focus Move Relative" {
          }
        }
        n494 = property on="Tab Control" class="TabCtl (strict)"("Val(Sgnl)"=w735) -> ()  [unwired: 2 in, 2 out]
      }
      event "Script": Value Change {
        (unwired) T38."Focus Motors" ("Tab Control")
        n495 = event-data() -> ("NewVal"=w796:i32)  [unwired: 1 in]
        n496 = Unbundle By Name(w792) -> ("state"=w790:refnum<user-event>, "Script"=w799:T20[])
        n497 = Index Array(array=w799, index=w796) -> (element=w795:T20)
        n498 = Unbundle By Name(w795) -> ("Action"=w794:T21, "Data"=w793:variant)
        n499 = Build Array(w795) -> (w798:T20[])
        n500 = call "CC Generate Script Text.vi"("Script"=w798) -> ("Script String"=w797:string)  [unwired: 9 in, 1 out]
        n501 = case shown="\"Define Object\"" w794 {
          tunnel: w793 -> [_ w810 w819 w828 w833 w838 w844 w853 w860 w864 w871 w877 w882 _ w890 w899]
          tunnel: w792 -> [w801 w806 w816 w825 w830 w835 w845 w854 w861 w865 w872 w878 w883 w885 w887 w898]
          tunnel: [w801 w805 w815 w824 w830 w835 w845 w854 w861 w865 w872 w878 w883 w885 w887 w898] -> w791
          tunnel: w790 -> [_ w804 w814 w823 _ _ _ _ _ _ _ _ _ _ _ _]
          tunnel: [w800 T38."Object" ("Tab Control") T38."Dithering" ("Tab Control") T38."Dithering" ("Tab Control") T38."Exposure" ("Tab Control") T38."Acquire" ("Tab Control") T38."Filter Wheel" ("Tab Control") T38."Focus Motors" ("Tab Control") T38."Focus Motors" ("Tab Control") T38."Focus Motors" ("Tab Control") T38."Macro" ("Tab Control") T38."Pause" ("Tab Control") T38."Ask" ("Tab Control") T38."Telescope" ("Tab Control") T38."Telescope" ("Tab Control") T38."Telescope" ("Tab Control")] -> w789
          frame "Noop", Default {
            n502 = property on="Tab Control" class="TabCtl (strict)"() -> ("Value"=w800:T1)  [unwired: 2 in, 2 out]
          }
          frame "Define Object" {
            n503 = Variant To Data(type=T14 {"Object"={"Name"=""}, "Sidereal Rate"={"dRA"=0.0, "dDEC"=0.0}, "RA and DEC"={"RA"=0.0, "DEC"=0.0}, "Proper Motion"={"muRA"=0.0, "muDEC"=0.0, "Epoch"=0.0}, "Offsets"={"RA"=0.0, "DEC"=0.0, "ROT"=0.0}, "Equinox"={"Equinox Year"=2000, "Equinox Prefix"="J"}, "Parallax"={"Parallax"=0.0, "rv kps"=0.0}, "Rotator"={"Frame"="", "PA"=0.0}, "Frame"=enum."FK5", "Frac Rate"=1.0, "Wavelength"=0.5} ("Object"), Variant=w810) -> (data=w808:T14)  [unwired: 1 in, 1 out]
            n504 = Unbundle By Name(w808) -> ("Object.Name"=w807:string)
            n505 = Generate User Event(user event=w804, event data cluster="show object" ("event data")) -> ()  [unwired: 2 in, 2 out]
            n506 = Bundle By Name(cluster=w806, "curr object"=w807) -> (w805:T26)
          }
          frame "Define Dithering" {
            n507 = Variant To Data(type=T9 {"Name"="", "Dithering Offsets"={"Offsets"=[]}} ("Dithering Offsets"), Variant=w819) -> (data=w818:T9)  [unwired: 1 in, 1 out]
            n508 = Unbundle By Name(w818) -> ("Name"=w817:string)
            n509 = Generate User Event(user event=w814, event data cluster="show dither" ("event data")) -> ()  [unwired: 2 in, 2 out]
            n510 = Bundle By Name(cluster=w816, "curr object"=w817) -> (w815:T26)
          }
          frame "Define Random Dither" {
            n511 = Variant To Data(type=T8 {"Count"=1, "Radius"=1.0, "Name"=""} ("Dithering Offsets"), Variant=w828) -> (data=w827:T8)  [unwired: 1 in, 1 out]
            n512 = Unbundle By Name(w827) -> ("Name"=w826:string)
            n513 = Generate User Event(user event=w823, event data cluster="show dither" ("event data")) -> ()  [unwired: 2 in, 2 out]
            n514 = Bundle By Name(cluster=w825, "curr object"=w826) -> (w824:T26)
          }
          frame "Define Exposure" {
            n515 = Variant To Data(type=T6 {"Mode"=enum."CDS", "Integration Time"=1.0, "Name"="", "Images"=1} ("Exposure"), Variant=w833) -> (data=w831:T6)  [unwired: 1 in, 1 out]
            n516 = property on="Exposure" class="Clust (strict)"("Value"=w831) -> ()  [unwired: 2 in, 2 out]
          }
          frame "Acquire Images" {
            n517 = Variant To Data(type=T35 {"Object"="", "Exposure"="", "Dithering"=""} ("Acquire Parameters"), Variant=w838) -> (data=w836:T35)  [unwired: 1 in, 1 out]
            n518 = property on="Acquire Parameters" class="Clust (strict)"("Value"=w836) -> ()  [unwired: 2 in, 2 out]
          }
          frame "Set Filter Wheel" {
            (unwired) T51."Filter Wheel" ("Tab Control")
            n519 = Variant To Data(type=T32 {"Wheel"=0, "Filter"=0} ("Acquire Parameters"), Variant=w844) -> (data=w842:T32)  [unwired: 1 in, 1 out]
            n520 = Unbundle By Name(w842) -> ("Wheel"=w841:i32, "Filter"=w840:i32)
            n521 = case shown="0, Default" w841 {
              tunnel: w840 -> [w846 w847]
              frame 0, Default {
                n522 = property on="Filter Wheel 1" class="LstBox (strict)"("Value"=w846) -> ()  [unwired: 2 in, 2 out]
              }
              frame 1 {
                n523 = property on="Filter Wheel 2" class="LstBox (strict)"("Value"=w847) -> ()  [unwired: 2 in, 2 out]
              }
            }
          }
          frame "Focus Move Relative" {
            n524 = Variant To Data(type=T30 {"Motor"=0, "Position"=0}, Variant=w853) -> (data=w850:T30)  [unwired: 1 in, 1 out]
            n525 = Unbundle By Name(w850) -> ("Motor"=w849:i32, "Position"=w848:i32)
            n526 = local write "Select Motor (0:n-1)"(w849) -> ()
            n527 = local write "Steps"(w848) -> ()
          }
          frame "Focus Move Absolute" {
            n528 = Variant To Data(type=T30 {"Motor"=0, "Position"=0} ("Cluster"), Variant=w860) -> (data=w858:T30)  [unwired: 1 in, 1 out]
            n529 = Unbundle By Name(w858) -> ("Motor"=w857:i32, "Position"=w856:i32)
            n530 = local write "Select Motor (0:n-1)"(w857) -> ()
            n531 = local write "Steps"(w856) -> ()
          }
          frame "Focus Set Home" {
            n532 = Variant To Data(type=0, Variant=w864) -> ()  [unwired: 1 in, 2 out]
          }
          frame "Macro" {
            n533 = Variant To Data(type="", Variant=w871) -> (data=w868:string)  [unwired: 1 in, 1 out]
            n534 = property on="Script to Call" class="Ring (strict)"() -> ("Strings []"=w869:string[])  [unwired: 2 in, 2 out]
            n535 = Search 1D Array(1D array=w869, element=w868) -> (index of element=w867:i32)  [unwired: 1 in]
            n536 = property on="Script to Call" class="Ring (strict)"("Value"=w867) -> ()  [unwired: 2 in, 2 out]
          }
          frame "Pause" {
            n537 = Variant To Data(type=T37 {"Time (s)"=0.0} ("Pause Parameters"), Variant=w877) -> (data=w876:T37)  [unwired: 1 in, 1 out]
            n538 = Unbundle By Name(w876) -> ("Time (s)"=w874:dbl)
            n539 = local write "Seconds to Pause"(w874) -> ()
          }
          frame "Ask User" {
            n540 = Variant To Data(type="", Variant=w882) -> (data=w880:string)  [unwired: 1 in, 1 out]
            n541 = local write "Message for User"(w880) -> ()
          }
          frame "Telescope Home" {
          }
          frame "Telescope Move" {
            n542 = Variant To Data(type=0.0, Variant=w890) -> (data=w888:dbl)  [unwired: 1 in, 1 out]
            n543 = property on="Position" class="DigNum (strict)"("Value"=w888) -> ()  [unwired: 2 in, 2 out]
          }
          frame "Telescope RA DEC" {
            n544 = Variant To Data(type=T15 {"RA"=0.0, "DEC"=0.0} ("Position"), Variant=w899) -> (data=w896:T15)  [unwired: 1 in, 1 out]
            n545 = call "CC Convert RA and DEC to HHMMSS.vi"("RA and DEC"=w896) -> ("DEC String"=w893:string, "RA String"=w894:string)  [unwired: 7 in, 2 out]
            n546 = Bundle(cluster=cluster{"RA":string, "DEC":string} {"RA"="02:22:00.0", "DEC"="24:55:00.0"} ("RA and DEC String 2"), "RA"=w894, "DEC"=w893) -> (w892:cluster{"RA":string, "DEC":string})
            n547 = property on="RA and DEC String 2" class="Clust (strict)"("Value"=w892) -> ()  [unwired: 2 in, 2 out]
          }
        }
        n548 = property on="Script Line" class="Str"("Value"=w797) -> ()  [unwired: 2 in, 2 out]
        n549 = property on="Tab Control" class="TabCtl (strict)"("Value"=w789) -> ()  [unwired: 2 in, 2 out]
      }
      event "Send": Value Change {
        n550 = event-data() -> ()  [unwired: 1 in, 6 out]
        n551 = call "CC Script Parse.vi"("Script text"="Script Line") -> ("Syntax Errors"=w900:string, "Script Ok?"=w903:bool, "Script steps"=w904:T20[])  [unwired: 7 in, 1 out]
        n552 = case shown="True" w903 {
          tunnel: w904 -> [_ w914]
          tunnel: w901 -> [w909 w912]
          tunnel: [w909 w913] -> w902
          tunnel: w900 -> [w907 _]
          frame False {
            n553 = Format Into String(format string="Error in script line: %s", w907) -> (resulting string=w906:string)  [unwired: 2 in, 1 out]
            n554 = One Button Dialog(message=w906) -> ()  [unwired: 1 in, 1 out]
          }
          frame True {
            n555 = Bundle By Name(cluster=w912, "test"=w914) -> (w913:T26)
            n556 = Unbundle By Name(w912) -> ("state"=w911:refnum<user-event>)
            n557 = Generate User Event(user event=w911, event data cluster="run test" ("event data")) -> ()  [unwired: 2 in, 2 out]
          }
        }
      }
      event "Add Ask": Value Change {
        n558 = event-data() -> ()  [unwired: 1 in, 1 out]
        n559 = Unbundle By Name(w915) -> ("Script"=w922:T20[], "state"=w919:refnum<user-event>)
        n560 = Generate User Event(user event=w919, event data cluster="update script" ("event data")) -> ()  [unwired: 2 in, 2 out]
        n561 = Bundle By Name(cluster=T20 {"Action"=enum."Acquire Images", "Data"=variant}, "Action"=CC_enum_Script_Action."Ask User", "Data"="Message for User") -> (w921:T20)
        n562 = Build Array (concatenate)(w922, w921) -> (w920:T20[])
        n563 = Bundle By Name(cluster=w915, "Script"=w920) -> (w916:T26)
      }
      event "Add CmdLine": Value Change {
        n564 = event-data() -> ()  [unwired: 1 in, 1 out]
        n565 = Unbundle By Name(w926) -> ("Script"=w932:T20[], "state"=w929:refnum<user-event>)
        n566 = Generate User Event(user event=w929, event data cluster="update script" ("event data")) -> ()  [unwired: 2 in, 2 out]
        n567 = Bundle By Name(cluster=T20 {"Action"=enum."Acquire Images", "Data"=variant}, "Action"=CC_enum_Script_Action."CmdLine", "Data"="Command Line") -> (w931:T20)
        n568 = Build Array (concatenate)(w932, w931) -> (w930:T20[])
        n569 = Bundle By Name(cluster=w926, "Script"=w930) -> (w927:T26)
      }
      event "Add Macro": Value Change {
        n570 = event-data() -> ()  [unwired: 1 in, 1 out]
        n571 = property on="Script to Call" class="Ring (strict)"() -> ("Strings []"=w937:string[])  [unwired: 2 in, 2 out]
        n572 = Unbundle By Name(w938) -> ("Script"=w944:T20[], "state"=w941:refnum<user-event>)
        n573 = Index Array(array=w937, index="Script to Call") -> (element=w935:string)
        n574 = Generate User Event(user event=w941, event data cluster="update script" ("event data")) -> ()  [unwired: 2 in, 2 out]
        n575 = Bundle By Name(cluster=T20 {"Action"=enum."Acquire Images", "Data"=variant}, "Action"=CC_enum_Script_Action."Macro", "Data"=w935) -> (w943:T20)
        n576 = Build Array (concatenate)(w944, w943) -> (w942:T20[])
        n577 = Bundle By Name(cluster=w938, "Script"=w942) -> (w939:T26)
      }
      event "Add No-op": Value Change {
        n578 = event-data() -> ()  [unwired: 1 in, 1 out]
        n579 = Unbundle By Name(w947) -> ("Script"=w953:T20[], "state"=w950:refnum<user-event>)
        n580 = Generate User Event(user event=w950, event data cluster="update script" ("event data")) -> ()  [unwired: 2 in, 2 out]
        n581 = Bundle By Name(cluster=T20 {"Action"=enum."Acquire Images", "Data"=variant}, "Action"=CC_enum_Script_Action."Noop") -> (w952:T20)
        n582 = Build Array (concatenate)(w953, w952) -> (w951:T20[])
        n583 = Bundle By Name(cluster=w947, "Script"=w951) -> (w948:T26)
      }
      event "Add Pause": Value Change {
        n584 = event-data() -> ()  [unwired: 1 in, 1 out]
        n585 = Unbundle By Name(w959) -> ("Script"=w965:T20[], "state"=w962:refnum<user-event>)
        n586 = Bundle By Name(cluster=T37 {"Time (s)"=0.0} ("Pause Parameters"), "Time (s)"="Seconds to Pause") -> (w957:T37)
        n587 = Generate User Event(user event=w962, event data cluster="update script" ("event data")) -> ()  [unwired: 2 in, 2 out]
        n588 = Bundle By Name(cluster=T20 {"Action"=enum."Acquire Images", "Data"=variant}, "Action"=CC_enum_Script_Action."Pause", "Data"=w957) -> (w964:T20)
        n589 = Build Array (concatenate)(w965, w964) -> (w963:T20[])
        n590 = Bundle By Name(cluster=w959, "Script"=w963) -> (w960:T26)
      }
      event "Script": Shortcut Menu Activation? {
        n591 = event-data() -> ("CtlRef"=w973:refnum<vi>, "Coords"=w972:T48)  [unwired: 1 in]
        n592 = invoke class="MCListbox (strict)" method="Point To Row Column"(reference=w973, "Point"=w972) -> ("InBounds"=w970:bool, "CellPosition"=w971:T49)  [unwired: 5 in, 5 out]
        n593 = Unbundle By Name(w971) -> ("Row"=w968:i32)
        n594 = property on="Script" class="MCListbox (strict)"("Value"=w968) -> ()  [unwired: 2 in, 2 out]
        n595 = Not(x=w970) -> (.not. x?=w969:bool)
        n596 = event-data("Discard?"=w969) -> ()  [unwired: 1 in, 1 out]
      }
      event "Script": Shortcut Menu Selection (User) {
        n597 = event-data() -> ("CtlRef"=w980:refnum<vi>, "ItemTag"=w981:string)  [unwired: 1 in, 3 out]
        n598 = property class="MCListbox (strict)"(reference=w980) -> ("Value"=w978:i32)  [unwired: 1 in, 2 out]
        n599 = Unbundle By Name(w976) -> ("state"=w977:refnum<user-event>, "Script"=w979:T20[])
        n600 = case shown="\"Delete Step\"" w981 {
          tunnel: w979 -> [_ w984 w995 w1003]
          tunnel: w978 -> [_ w987 w994 w1002]
          tunnel: w977 -> [_ w992 w1000 w1008]
          tunnel: w976 -> [w982 w990 w998 w1006]
          tunnel: [w982 w988 w997 w1005] -> w975
          frame "False", Default {
          }
          frame "Delete Step" {
            n601 = Delete From Array(array=w984, index=w987) -> (array with subset deleted=w989:T20[])  [unwired: 1 in, 1 out]
            n602 = Array Size(array=w984) -> (size(s)=w985:i32)
            n603 = In Range and Coerce(upper limit=w985, x=w987, lower limit=0) -> (coerced(x)=w983:i32)  [unwired: 1 out]
            n604 = Bundle By Name(cluster=w990, "Script"=w989) -> (w988:T26)
            n605 = property on="Script" class="MCListbox (strict)"("Value"=w983) -> ()  [unwired: 2 in, 2 out]
            n606 = Generate User Event(user event=w992, event data cluster="update script" ("event data")) -> ()  [unwired: 2 in, 2 out]
          }
          frame "Move Down" {
            n607 = Increment(x=w994) -> (x+1=w993:i32)
            n608 = Generate User Event(user event=w1000, event data cluster="update script" ("event data")) -> ()  [unwired: 2 in, 2 out]
            n609 = call "CC Swap Script Steps.vi"("index"=w994, "Script in"=w995) -> ("Script out"=w996:T20[])  [unwired: 8 in, 1 out]
            n610 = property on="Script" class="MCListbox (strict)"("Value"=w993) -> ()  [unwired: 2 in, 2 out]
            n611 = Bundle By Name(cluster=w998, "Script"=w996) -> (w997:T26)
          }
          frame "Move Up" {
            n612 = Decrement(x=w1002) -> (x-1=w1001:i32)
            n613 = Generate User Event(user event=w1008, event data cluster="update script" ("event data")) -> ()  [unwired: 2 in, 2 out]
            n614 = call "CC Swap Script Steps.vi"("index"=w1001, "Script in"=w1003) -> ("Script out"=w1004:T20[])  [unwired: 8 in, 1 out]
            n615 = property on="Script" class="MCListbox (strict)"("Value"=w1001) -> ()  [unwired: 2 in, 2 out]
            n616 = Bundle By Name(cluster=w1006, "Script"=w1004) -> (w1005:T26)
          }
        }
      }
      event "Script": Shortcut Menu Selection? (App) {
        n617 = event-data() -> ()  [unwired: 1 in, 8 out]
        n618 = event-data("Discard?"=FALSE) -> ()  [unwired: 1 in, 1 out]
      }
      event "Close": Value Change {
        n619 = event-data() -> ()  [unwired: 1 in, 1 out]
        n620 = Unbundle By Name(w1014) -> ("Settings"=w1012:T22)
        n621 = Unbundle By Name(w1012) -> ("Script"=→"script name out":string)
        n622 = call "Rd Wr Script Defaults.vi"("Write? (F:Read)"=TRUE, "Script Settings"=w1012) -> ()  [unwired: 8 in, 2 out]
      }
    }
  }
